vi "Log_heading-replay_v1.vi"() -> ()   [LabVIEW 2019]
panel:
  out "2D Picture 2":picture
  in  "file path":path
  out "Waveform Graph":dbl[](graph)
  out "array":dbl[](array[numeric])
  out "wgs84 graph":cluster{"X":dbl, "Y":dbl}[](graph)=[{"X"=4531061.36242506, "Y"=6178441.986275759}, {"X"=4531061.095248447, "Y"=6178442.06681065}, {"X"=4531060.929819513, "Y"=6178442.13471346}, {"X"=4531060.832518823, "Y"=6178442.197541265}, {"X"=4531060.770616335, "Y"=6178442.272890285}, {"X"=4531060.789204832, "Y"=6178442.28919004}, {"X"=4531060.772395123, "Y"=6178442.292968577}, {"X"=4531060.722855385, "Y"=6178442.314343328}, {"X"=4531060.606076811, "Y"=6178442.350832218}, {"X"=4531060.439758502, "Y"=6178442.40869586}, {"X"=4531060.290249909, "Y"=6178442.462780965}, {"X"=4531060.272550807, "Y"=6178442.456520356}, {"X"=4531060.239820785, "Y"=6178442.474116567}, {"X"=4531060.192059842, "Y"=6178442.5155695975}, {"X"=4531059.864759631, "Y"=6178442.691531702}, {"X"=4531059.779821708, "Y"=6178442.700385227}, {"X"=4531059.660374976, "Y"=6178442.7067566775}, {"X"=4531059.540038856, "Y"=6178442.7030889895}, {"X"=4531059.436512438, "Y"=6178442.695642762}, {"X"=4531059.299366613, "Y"=6178442.695753609}, {"X"=4531059.242711737, "Y"=6178442.6368152285}, {"X"=4531059.155105636, "Y"=6178442.615551336}, {"X"=4531059.104676525, "Y"=6178442.626886936}, {"X"=4531059.137406536, "Y"=6178442.609290733}, {"X"=4531059.171025946, "Y"=6178442.601733663}, {"X"=4531059.187835644, "Y"=6178442.597955129}, {"X"=4531059.189614435, "Y"=6178442.618033409}, {"X"=4531059.194950805, "Y"=6178442.678268249}, {"X"=4531059.527676117, "Y"=6178442.757063225}, {"X"=4531059.803746564, "Y"=6178442.776919831}, {"X"=4531059.710892868, "Y"=6178442.889943297}, {"X"=4531059.54190642, "Y"=6178442.917689476}, {"X"=4531059.377366953, "Y"=6178442.995631349}, {"X"=4531059.319911462, "Y"=6178443.121176009}, {"X"=4531058.873164632, "Y"=6178443.303509431}, {"X"=4531058.264546617, "Y"=6178443.593902031}, {"X"=4531057.714273541, "Y"=6178443.768789094}, {"X"=4531056.857868471, "Y"=6178443.971533049}, {"X"=4531055.882016951, "Y"=6178444.180648344}, {"X"=4531054.316047871, "Y"=6178444.501933605}, {"X"=4531053.000445728, "Y"=6178444.746462661}, {"X"=4531051.687423223, "Y"=6178444.826587329}, {"X"=4531050.336334684, "Y"=6178444.864073566}, {"X"=4531049.315213942, "Y"=6178444.755715789}, {"X"=4531048.093266786, "Y"=6178444.702739513}, {"X"=4531047.005797124, "Y"=6178444.619535221}, {"X"=4531046.041331673, "Y"=6178444.570115978}, {"X"=4531045.022790559, "Y"=6178444.297354844}, {"X"=4531044.25817308, "Y"=6178443.987994255}, {"X"=4531042.963740925, "Y"=6178444.084419535}, {"X"=4531041.977219151, "Y"=6178444.173065893}, {"X"=4531040.82438002, "Y"=6178444.319575647}, {"X"=4531039.649394999, "Y"=6178444.409629484}, {"X"=4531038.509808348, "Y"=6178444.512204443}, {"X"=4531037.261359377, "Y"=6178444.547098991}, {"X"=4531036.311926155, "Y"=6178444.473824003}, {"X"=4531035.260745918, "Y"=6178444.41318121}, {"X"=4531033.905213919, "Y"=6178444.400473842}, {"X"=4531032.472749636, "Y"=6178444.486971602}, {"X"=4531031.387061386, "Y"=6178444.423847185}, {"X"=4531030.066928328, "Y"=6178444.42366126}, {"X"=4531029.049278559, "Y"=6178444.16094189}, {"X"=4531027.591021638, "Y"=6178443.95630831}, {"X"=4531026.079757724, "Y"=6178443.927413569}, {"X"=4531024.871066671, "Y"=6178443.830505573}, {"X"=4531023.563297236, "Y"=6178443.77634695}, {"X"=4531022.521812914, "Y"=6178443.631615039}, {"X"=4531021.367998429, "Y"=6178443.573567053}, {"X"=4531020.007132588, "Y"=6178443.500627522}, {"X"=4531018.452557386, "Y"=6178443.563381526}, {"X"=4531016.914792171, "Y"=6178443.622357118}, {"X"=4531015.791039957, "Y"=6178443.516596719}, {"X"=4531014.692901826, "Y"=6178443.312928568}, {"X"=4531013.452372559, "Y"=6178443.243657234}, {"X"=4531012.218959265, "Y"=6178443.2546979}, {"X"=4531010.736961054, "Y"=6178443.362572499}, {"X"=4531009.554067381, "Y"=6178443.556796684}, {"X"=4531008.330439165, "Y"=6178443.678266158}, {"X"=4531007.172270388, "Y"=6178443.764543629}, {"X"=4531006.182197059, "Y"=6178443.813035869}, {"X"=4531004.925749518, "Y"=6178443.757582804}, {"X"=4531003.509212434, "Y"=6178443.830265695}, {"X"=4531002.303193948, "Y"=6178443.763477351}, {"X"=4531001.0052135065, "Y"=6178443.819749711}, {"X"=4530999.847845012, "Y"=6178443.721548208}, {"X"=4530998.599222504, "Y"=6178443.367409869}, {"X"=4530997.372746514, "Y"=6178443.069726953}, {"X"=4530996.291420466, "Y"=6178442.862283204}, {"X"=4530995.270216481, "Y"=6178442.559414194}, {"X"=4530994.338396943, "Y"=6178442.297886271}, {"X"=4530993.687891098, "Y"=6178441.921928868}, {"X"=4530993.020575724, "Y"=6178441.549750173}, {"X"=4530992.446202746, "Y"=6178441.259068059}, {"X"=4530991.660331448, "Y"=6178440.903300595}, {"X"=4530990.862987714, "Y"=6178440.61154533}, {"X"=4530989.863930333, "Y"=6178440.365132826}, {"X"=4530988.785181954, "Y"=6178439.993290142}, {"X"=4530987.896674796, "Y"=6178439.640117105}, {"X"=4530987.016081899, "Y"=6178439.182776809}, {"X"=4530986.158525055, "Y"=6178438.791930499}, {"X"=4530985.322133756, "Y"=6178438.252982851}, {"X"=4530984.685768332, "Y"=6178437.843132436}, {"X"=4530984.103297727, "Y"=6178437.267584608}, {"X"=4530983.746466159, "Y"=6178436.723226662}, {"X"=4530983.743430932, "Y"=6178435.915040186}, {"X"=4530983.693525295, "Y"=6178435.158344908}, {"X"=4530983.556014049, "Y"=6178434.380386928}, {"X"=4530983.381325537, "Y"=6178433.569830535}, {"X"=4530983.004923267, "Y"=6178432.804617277}, {"X"=4530982.739960196, "Y"=6178431.942681698}, {"X"=4530982.790020886, "Y"=6178431.1532757515}, {"X"=4530982.649042446, "Y"=6178430.529679693}, {"X"=4530982.459322566, "Y"=6178429.742979693}, {"X"=4530982.320920433, "Y"=6178428.954982738}, {"X"=4530982.173622549, "Y"=6178428.0665968135}, {"X"=4530981.62823454, "Y"=6178427.329131322}, {"X"=4530981.438513815, "Y"=6178426.54243141}, {"X"=4530981.246124193, "Y"=6178425.725614818}, {"X"=4530981.223608197, "Y"=6178424.89108958}, {"X"=4530981.094100545, "Y"=6178424.203481528}, {"X"=4530980.915053897, "Y"=6178423.537248316}, {"X"=4530981.074865304, "Y"=6178422.825558664}, {"X"=4530981.669943885, "Y"=6178421.995545852}, {"X"=4530981.934170355, "Y"=6178421.301339371}, {"X"=4530982.416030478, "Y"=6178420.547971078}, {"X"=4530982.20603299, "Y"=6178419.919411453}, {"X"=4530982.59761853, "Y"=6178419.114663753}, {"X"=4530982.943223482, "Y"=6178418.371446361}, {"X"=4530983.023434869, "Y"=6178417.7288433835}, {"X"=4530983.0691375965, "Y"=6178417.083758783}, {"X"=4530983.532501486, "Y"=6178416.508607976}, {"X"=4530984.062121182, "Y"=6178415.71378513}, {"X"=4530984.575728308, "Y"=6178414.738261373}, {"X"=4530985.043354852, "Y"=6178413.824267901}, {"X"=4530985.719812219, "Y"=6178412.945240799}, {"X"=4530986.349399512, "Y"=6178412.117705096}, {"X"=4530986.909969615, "Y"=6178411.285206017}, {"X"=4530987.637838169, "Y"=6178410.5993987685}, {"X"=4530988.845269547, "Y"=6178409.908175884}, {"X"=4530990.169478464, "Y"=6178409.180462327}, {"X"=4530991.561908379, "Y"=6178408.642190958}, {"X"=4530992.899369467, "Y"=6178407.87054172}, {"X"=4530993.945731143, "Y"=6178407.102896896}, {"X"=4530995.245126048, "Y"=6178406.288609087}, {"X"=4530996.648047593, "Y"=6178405.481764915}, {"X"=4530997.913824367, "Y"=6178404.675033256}, {"X"=4530998.862888482, "Y"=6178403.970214601}, {"X"=4530999.767658552, "Y"=6178403.15248521}, {"X"=4531000.828163074, "Y"=6178402.350941164}, {"X"=4531001.817871174, "Y"=6178401.524355709}, {"X"=4531002.7430099705, "Y"=6178400.743001848}, {"X"=4531003.608027404, "Y"=6178400.057074705}, {"X"=4531004.825157088, "Y"=6178399.281753247}, {"X"=4531005.845816726, "Y"=6178398.41749089}, {"X"=4531006.73022056, "Y"=6178397.563380394}, {"X"=4531007.61640379, "Y"=6178396.729347373}, {"X"=4531008.417742332, "Y"=6178396.098689213}, {"X"=4531009.312821996, "Y"=6178395.365045503}, {"X"=4531010.308759668, "Y"=6178394.608728314}, {"X"=4531010.841941455, "Y"=6178393.854048861}, {"X"=4531011.543219663, "Y"=6178393.061580644}, {"X"=4531012.576335659, "Y"=6178392.337860493}, {"X"=4531013.4466002695, "Y"=6178391.517641876}, {"X"=4531014.00895371, "Y"=6178390.705207859}, {"X"=4531014.772226336, "Y"=6178390.031908954}, {"X"=4531015.669976403, "Y"=6178389.328378749}, {"X"=4531016.655240558, "Y"=6178388.451588911}, {"X"=4531017.595413627, "Y"=6178387.646369493}, {"X"=4531018.445404212, "Y"=6178386.9842916755}, {"X"=4531018.971563079, "Y"=6178386.343816914}, {"X"=4531019.59324242, "Y"=6178385.6204340765}, {"X"=4531020.280474299, "Y"=6178385.056378583}, {"X"=4531021.072029946, "Y"=6178384.315284261}, {"X"=4531021.529967807, "Y"=6178383.485363264}, {"X"=4531022.314406787, "Y"=6178382.663955374}, {"X"=4531023.2032625815, "Y"=6178381.860029902}, {"X"=4531024.23727163, "Y"=6178381.1463417495}, {"X"=4531024.742173449, "Y"=6178380.459447751}, {"X"=4531025.615999362, "Y"=6178379.679377978}, {"X"=4531026.621634371, "Y"=6178378.838958925}, {"X"=4531027.767974779, "Y"=6178378.038581567}, {"X"=4531028.709929959, "Y"=6178377.2534335395}, {"X"=4531029.719124331, "Y"=6178376.453169198}, {"X"=4531030.5036580935, "Y"=6178375.826279149}, {"X"=4531031.516411452, "Y"=6178375.066170328}, {"X"=4531032.342478642, "Y"=6178374.327551261}, {"X"=4531033.658790734, "Y"=6178373.7039818335}, {"X"=4531035.2352562575, "Y"=6178373.114079729}, {"X"=4531036.86571019, "Y"=6178372.552996834}, {"X"=4531038.35555227, "Y"=6178372.146394164}, {"X"=4531039.811775328, "Y"=6178371.747349183}, {"X"=4531041.074288043, "Y"=6178371.484004215}, {"X"=4531042.657966306, "Y"=6178371.168936872}, {"X"=4531043.966553982, "Y"=6178371.038582218}, {"X"=4531045.505234291, "Y"=6178370.989610227}, {"X"=4531046.940387374, "Y"=6178370.933194681}, {"X"=4531048.287043757, "Y"=6178370.845478166}, {"X"=4531049.462136587, "Y"=6178370.949918508}, {"X"=4531050.707137665, "Y"=6178371.069360725}, {"X"=4531051.925636092, "Y"=6178371.276674773}, {"X"=4531053.001649715, "Y"=6178371.423868022}, {"X"=4531054.063522423, "Y"=6178371.604958085}, {"X"=4531055.343923036, "Y"=6178371.73692166}, {"X"=4531056.731409991, "Y"=6178371.916486175}, {"X"=4531057.948130019, "Y"=6178372.103723062}, {"X"=4531059.2674884265, "Y"=6178372.288364829}, {"X"=4531060.41163191, "Y"=6178372.4304827275}, {"X"=4531061.5637817625, "Y"=6178372.662953975}, {"X"=4531062.82390746, "Y"=6178372.95306562}, {"X"=4531064.037069952, "Y"=6178373.100146859}, {"X"=4531065.249343056, "Y"=6178373.237189062}, {"X"=4531066.432444453, "Y"=6178373.4319857}, {"X"=4531067.647386592, "Y"=6178373.599146142}, {"X"=4531068.807543307, "Y"=6178373.921972353}, {"X"=4531069.985399526, "Y"=6178374.251059206}, {"X"=4531071.112826171, "Y"=6178374.591483286}, {"X"=4531072.362278149, "Y"=6178374.761126214}, {"X"=4531073.548938524, "Y"=6178374.996081617}, {"X"=4531074.734709472, "Y"=6178375.220998018}, {"X"=4531075.988518144, "Y"=6178375.2463128045}, {"X"=4531077.323799403, "Y"=6178375.417140541}, {"X"=4531078.632577418, "Y"=6178375.675840814}, {"X"=4531079.936018335, "Y"=6178375.874305648}, {"X"=4531081.3721596515, "Y"=6178376.0224605715}, {"X"=4531082.628729365, "Y"=6178376.27242007}, {"X"=4531083.877384625, "Y"=6178376.626551941}, {"X"=4531085.0180641785, "Y"=6178376.923043358}, {"X"=4531086.153406647, "Y"=6178377.159299181}, {"X"=4531086.974697717, "Y"=6178377.527591075}, {"X"=4531087.4545440385, "Y"=6178378.105752066}, {"X"=4531088.40141923, "Y"=6178378.343419691}, {"X"=4531089.834003558, "Y"=6178378.451419775}, {"X"=4531091.277262362, "Y"=6178378.67989211}, {"X"=4531092.574568948, "Y"=6178379.0026112255}, {"X"=4531093.840833539, "Y"=6178379.168480203}, {"X"=4531095.048662892, "Y"=6178379.25533212}, {"X"=4531095.938083443, "Y"=6178379.618549757}, {"X"=4531096.926584712, "Y"=6178379.939015398}, {"X"=4531098.373402462, "Y"=6178380.207647139}, {"X"=4531099.6042688675, "Y"=6178380.360996598}, {"X"=4531100.833356456, "Y"=6178380.494267572}, {"X"=4531102.114653141, "Y"=6178380.63628074}, {"X"=4531103.531319355, "Y"=6178380.758102154}, {"X"=4531104.69939403, "Y"=6178380.97676513}, {"X"=4531105.671885175, "Y"=6178381.116523916}, {"X"=4531106.82137114, "Y"=6178381.318887517}, {"X"=4531108.565433378, "Y"=6178381.45926503}, {"X"=4531110.451801206, "Y"=6178381.270711307}, {"X"=4531112.307218145, "Y"=6178381.119833651}, {"X"=4531114.310367992, "Y"=6178380.8947881535}, {"X"=4531116.179927931, "Y"=6178380.710013429}, {"X"=4531117.915008334, "Y"=6178380.555470101}, {"X"=4531119.4837679025, "Y"=6178380.458794905}, {"X"=4531121.222407262, "Y"=6178380.344409419}, {"X"=4531123.170683199, "Y"=6178380.080503614}, {"X"=4531124.669535756, "Y"=6178379.968825969}, {"X"=4531126.092343553, "Y"=6178379.966398067}, {"X"=4531127.391255065, "Y"=6178379.92014661}, {"X"=4531128.363659995, "Y"=6178379.865379146}, {"X"=4531129.900581387, "Y"=6178379.7963412525}, {"X"=4531131.0968544325, "Y"=6178379.752684653}, {"X"=4531132.079133352, "Y"=6178380.002880428}, {"X"=4531133.501053443, "Y"=6178379.990413857}, {"X"=4531134.7982770335, "Y"=6178380.118613123}, {"X"=4531135.797366396, "Y"=6178380.365030662}, {"X"=4531137.091032587, "Y"=6178380.453072453}, {"X"=4531138.366999476, "Y"=6178380.534853874}, {"X"=4531139.581952214, "Y"=6178380.702027647}, {"X"=4531140.701291988, "Y"=6178380.757582756}, {"X"=4531141.9710335145, "Y"=6178380.769088216}, {"X"=4531143.468201078, "Y"=6178380.831862938}, {"X"=4531145.047640736, "Y"=6178380.85566426}, {"X"=4531146.485484407, "Y"=6178380.829380992}, {"X"=4531148.187932283, "Y"=6178380.886967416}, {"X"=4531149.763815479, "Y"=6178380.870611242}, {"X"=4531150.981349615, "Y"=6178380.873375337}, {"X"=4531152.508581932, "Y"=6178380.888435311}, {"X"=4531154.135697515, "Y"=6178380.676252104}, {"X"=4531155.785938228, "Y"=6178380.725097228}, {"X"=4531158.006835585, "Y"=6178380.635419734}, {"X"=4531159.500449378, "Y"=6178380.658038273}, {"X"=4531160.778287833, "Y"=6178380.954432427}, {"X"=4531162.149872312, "Y"=6178381.147836851}, {"X"=4531163.841739914, "Y"=6178381.27948173}, {"X"=4531165.326637487, "Y"=6178381.59076749}, {"X"=4531166.717701023, "Y"=6178381.8105128035}, {"X"=4531168.529821052, "Y"=6178381.751294012}, {"X"=4531169.835055363, "Y"=6178381.969855328}, {"X"=4531170.320948598, "Y"=6178382.229250287}, {"X"=4531171.080252015, "Y"=6178382.478380797}, {"X"=4531171.576016277, "Y"=6178383.042742996}, {"X"=4531172.72035149, "Y"=6178383.573942711}, {"X"=4531174.0849103825, "Y"=6178383.88156489}, {"X"=4531175.150355192, "Y"=6178384.102834543}, {"X"=4531175.369952878, "Y"=6178384.452811636}, {"X"=4531175.2817180995, "Y"=6178385.005102757}, {"X"=4531174.792706191, "Y"=6178385.678205996}, {"X"=4531174.569187919, "Y"=6178386.445219818}, {"X"=4531173.566174453, "Y"=6178387.315784675}, {"X"=4531173.004585712, "Y"=6178387.943764852}, {"X"=4531172.677538117, "Y"=6178388.703332222}, {"X"=4531172.19386255, "Y"=6178389.436671552}, {"X"=4531171.71018701, "Y"=6178390.170010573}, {"X"=4531171.741401999, "Y"=6178390.715927548}, {"X"=4531171.907987807, "Y"=6178391.2416532375}, {"X"=4531171.572046452, "Y"=6178391.90082367}, {"X"=4531171.167085634, "Y"=6178392.555030101}, {"X"=4531171.157652611, "Y"=6178393.222718802}, {"X"=4531170.708486615, "Y"=6178393.958538462}, {"X"=4531169.790414286, "Y"=6178394.820244326}, {"X"=4531169.3456951305, "Y"=6178395.606261164}, {"X"=4531168.858462186, "Y"=6178396.299439562}, {"X"=4531168.570283294, "Y"=6178396.917153108}, {"X"=4531168.074244299, "Y"=6178397.70446596}, {"X"=4531167.710907955, "Y"=6178398.441468852}, {"X"=4531167.532396106, "Y"=6178398.942374006}, {"X"=4531167.076115536, "Y"=6178399.597874829}, {"X"=4531166.6110288715, "Y"=6178400.347510266}, {"X"=4531166.296344272, "Y"=6178401.053096698}, {"X"=4531165.944482004, "Y"=6178401.726082247}, {"X"=4531165.362526449, "Y"=6178402.317677534}, {"X"=4531164.53900361, "Y"=6178402.891898637}, {"X"=4531163.9013690315, "Y"=6178403.629122646}, {"X"=4531163.401685826, "Y"=6178404.181744099}, {"X"=4531163.1179536, "Y"=6178404.849652828}, {"X"=4531162.782901618, "Y"=6178405.518858123}, {"X"=4531162.6849701125, "Y"=6178406.155239621}, {"X"=4531162.467588969, "Y"=6178406.7979932325}, {"X"=4531161.8820765605, "Y"=6178407.349428364}, {"X"=4531161.4178794585, "Y"=6178408.109100074}, {"X"=4531161.144818966, "Y"=6178408.897482027}, {"X"=4531160.637306067, "Y"=6178409.748805623}, {"X"=4531159.989976334, "Y"=6178410.570121538}, {"X"=4531159.336421459, "Y"=6178411.321160347}, {"X"=4531158.668724526, "Y"=6178412.10609606}, {"X"=4531158.485939669, "Y"=6178412.9458595095}, {"X"=4531157.989901085, "Y"=6178413.733165388}, {"X"=4531157.419594476, "Y"=6178414.6497991355}, {"X"=4531157.043894533, "Y"=6178415.440771885}, {"X"=4531156.463892334, "Y"=6178416.441499566}, {"X"=4531155.611371523, "Y"=6178417.462527762}, {"X"=4531155.200359533, "Y"=6178418.435506958}, {"X"=4531154.830884667, "Y"=6178419.296754719}, {"X"=4531154.30211532, "Y"=6178420.101654765}, {"X"=4531153.473432615, "Y"=6178421.004688968}, {"X"=4531152.974726329, "Y"=6178421.761872893}, {"X"=4531152.53801116, "Y"=6178422.638233842}, {"X"=4531152.18712486, "Y"=6178423.515780127}, {"X"=4531151.659244953, "Y"=6178424.330717752}, {"X"=4531150.965932405, "Y"=6178425.21355987}, {"X"=4531150.225746978, "Y"=6178426.1478953}, {"X"=4531149.141357127, "Y"=6178427.067447557}, {"X"=4531148.517953012, "Y"=6178427.965291934}, {"X"=4531147.82019449, "Y"=6178428.797934613}, {"X"=4531147.213600552, "Y"=6178429.691999431}, {"X"=4531146.807837723, "Y"=6178430.5306810085}, {"X"=4531146.549005081, "Y"=6178431.4796857955}, {"X"=4531146.207814394, "Y"=6178432.27313397}, {"X"=4531145.821442939, "Y"=6178432.943626221}, {"X"=4531145.026295356, "Y"=6178433.644567707}, {"X"=4531144.401112979, "Y"=6178434.522329833}, {"X"=4531143.8157756375, "Y"=6178435.462810415}, {"X"=4531142.856085532, "Y"=6178436.241694084}, {"X"=4531141.712202374, "Y"=6178436.683125389}, {"X"=4531140.460345346, "Y"=6178437.066912421}, {"X"=4531138.7855711365, "Y"=6178437.515045113}, {"X"=4531137.2540838905, "Y"=6178437.8388156835}, {"X"=4531135.901281937, "Y"=6178438.050746028}, {"X"=4531134.513081851, "Y"=6178438.250154628}, {"X"=4531133.302677512, "Y"=6178438.327683812}, {"X"=4531131.97727157, "Y"=6178438.461781153}, {"X"=4531130.434225819, "Y"=6178438.655039164}, {"X"=4531128.833636347, "Y"=6178438.779317742}, {"X"=4531127.188842603, "Y"=6178438.985207698}, {"X"=4531125.765159796, "Y"=6178438.977567875}, {"X"=4531124.333560398, "Y"=6178439.074100451}, {"X"=4531123.178034697, "Y"=6178439.19049111}, {"X"=4531121.688891792, "Y"=6178439.218044568}, {"X"=4531120.143983659, "Y"=6178439.196697701}, {"X"=4531118.777846783, "Y"=6178439.258037677}, {"X"=4531117.273760713, "Y"=6178439.503974881}, {"X"=4531115.719158377, "Y"=6178439.566721672}, {"X"=4531114.359247835, "Y"=6178439.698337167}, {"X"=4531112.978970496, "Y"=6178439.793573919}, {"X"=4531111.604831579, "Y"=6178439.764560291}, {"X"=4531110.167010706, "Y"=6178439.790818312}, {"X"=4531108.717716249, "Y"=6178439.881090899}, {"X"=4531107.251612302, "Y"=6178439.975142099}, {"X"=4531105.856218201, "Y"=6178439.899711062}, {"X"=4531104.335238762, "Y"=6178439.954901642}, {"X"=4531102.807232527, "Y"=6178440.124303117}, {"X"=4531101.328766988, "Y"=6178440.272329651}, {"X"=4531099.891838069, "Y"=6178440.308627729}, {"X"=4531098.531042268, "Y"=6178440.430204515}, {"X"=4531097.2551853685, "Y"=6178440.542927866}, {"X"=4531095.906753391, "Y"=6178440.610529815}, {"X"=4531094.453905393, "Y"=6178440.660646058}, {"X"=4531093.051487248, "Y"=6178440.699426771}, {"X"=4531091.507563893, "Y"=6178440.882646296}, {"X"=4531090.124624367, "Y"=6178440.947766378}, {"X"=4531088.636379567, "Y"=6178440.985361588}, {"X"=4531086.920802104, "Y"=6178441.166209676}, {"X"=4531085.168048208, "Y"=6178441.314457928}, {"X"=4531083.614256263, "Y"=6178441.1927222395}, {"X"=4531082.135708063, "Y"=6178441.1462256685}, {"X"=4531080.787191631, "Y"=6178441.019304884}, {"X"=4531079.550118306, "Y"=6178440.795660042}, {"X"=4531078.355558375, "Y"=6178440.664850496}, {"X"=4531077.03630355, "Y"=6178440.674700762}, {"X"=4531075.614411686, "Y"=6178440.68714403}, {"X"=4531074.112918239, "Y"=6178440.7686761385}, {"X"=4531072.594615453, "Y"=6178440.853986876}, {"X"=4531071.1807291135, "Y"=6178440.956783168}, {"X"=4531069.776626355, "Y"=6178441.170010469}, {"X"=4531068.367187707, "Y"=6178441.323002671}, {"X"=4531067.229284766, "Y"=6178441.251132974}, {"X"=4531066.229328779, "Y"=6178440.994669049}, {"X"=4531065.468266617, "Y"=6178440.725462372}, {"X"=4531065.011647067, "Y"=6178440.602842985}, {"X"=4531064.836523361, "Y"=6178440.754837769}, {"X"=4531064.734775603, "Y"=6178440.767469879}, {"X"=4531064.70204554, "Y"=6178440.7850661315}, {"X"=4531064.7259704, "Y"=6178440.861600875}, {"X"=4531064.616306829, "Y"=6178440.978403134}, {"X"=4531064.571213997, "Y"=6178441.049973729}, {"X"=4531064.4960592715, "Y"=6178441.16925804}, {"X"=4531064.430599156, "Y"=6178441.204450528}, {"X"=4531064.349218701, "Y"=6178441.253460727}, {"X"=4531064.235997578, "Y"=6178441.330106311}, {"X"=4531064.123665855, "Y"=6178441.41679105}, {"X"=4531064.026365073, "Y"=6178441.479618935}, {"X"=4531064.015781082, "Y"=6178441.553671578}, {"X"=4531064.05562626, "Y"=6178441.616388603}]
  in  "dt":u32=1
  out "utm graph":cluster{"X":dbl, "Y":dbl}[](graph)=[{"X"=4531061.36242506, "Y"=6178441.986275759}, {"X"=4531061.095248447, "Y"=6178442.06681065}, {"X"=4531060.929819513, "Y"=6178442.13471346}, {"X"=4531060.832518823, "Y"=6178442.197541265}, {"X"=4531060.770616335, "Y"=6178442.272890285}, {"X"=4531060.789204832, "Y"=6178442.28919004}, {"X"=4531060.772395123, "Y"=6178442.292968577}, {"X"=4531060.722855385, "Y"=6178442.314343328}, {"X"=4531060.606076811, "Y"=6178442.350832218}, {"X"=4531060.439758502, "Y"=6178442.40869586}, {"X"=4531060.290249909, "Y"=6178442.462780965}, {"X"=4531060.272550807, "Y"=6178442.456520356}, {"X"=4531060.239820785, "Y"=6178442.474116567}, {"X"=4531060.192059842, "Y"=6178442.5155695975}, {"X"=4531059.864759631, "Y"=6178442.691531702}, {"X"=4531059.779821708, "Y"=6178442.700385227}, {"X"=4531059.660374976, "Y"=6178442.7067566775}, {"X"=4531059.540038856, "Y"=6178442.7030889895}, {"X"=4531059.436512438, "Y"=6178442.695642762}, {"X"=4531059.299366613, "Y"=6178442.695753609}, {"X"=4531059.242711737, "Y"=6178442.6368152285}, {"X"=4531059.155105636, "Y"=6178442.615551336}, {"X"=4531059.104676525, "Y"=6178442.626886936}, {"X"=4531059.137406536, "Y"=6178442.609290733}, {"X"=4531059.171025946, "Y"=6178442.601733663}, {"X"=4531059.187835644, "Y"=6178442.597955129}, {"X"=4531059.189614435, "Y"=6178442.618033409}, {"X"=4531059.194950805, "Y"=6178442.678268249}, {"X"=4531059.527676117, "Y"=6178442.757063225}, {"X"=4531059.803746564, "Y"=6178442.776919831}, {"X"=4531059.710892868, "Y"=6178442.889943297}, {"X"=4531059.54190642, "Y"=6178442.917689476}, {"X"=4531059.377366953, "Y"=6178442.995631349}, {"X"=4531059.319911462, "Y"=6178443.121176009}, {"X"=4531058.873164632, "Y"=6178443.303509431}, {"X"=4531058.264546617, "Y"=6178443.593902031}, {"X"=4531057.714273541, "Y"=6178443.768789094}, {"X"=4531056.857868471, "Y"=6178443.971533049}, {"X"=4531055.882016951, "Y"=6178444.180648344}, {"X"=4531054.316047871, "Y"=6178444.501933605}, {"X"=4531053.000445728, "Y"=6178444.746462661}, {"X"=4531051.687423223, "Y"=6178444.826587329}, {"X"=4531050.336334684, "Y"=6178444.864073566}, {"X"=4531049.315213942, "Y"=6178444.755715789}, {"X"=4531048.093266786, "Y"=6178444.702739513}, {"X"=4531047.005797124, "Y"=6178444.619535221}, {"X"=4531046.041331673, "Y"=6178444.570115978}, {"X"=4531045.022790559, "Y"=6178444.297354844}, {"X"=4531044.25817308, "Y"=6178443.987994255}, {"X"=4531042.963740925, "Y"=6178444.084419535}, {"X"=4531041.977219151, "Y"=6178444.173065893}, {"X"=4531040.82438002, "Y"=6178444.319575647}, {"X"=4531039.649394999, "Y"=6178444.409629484}, {"X"=4531038.509808348, "Y"=6178444.512204443}, {"X"=4531037.261359377, "Y"=6178444.547098991}, {"X"=4531036.311926155, "Y"=6178444.473824003}, {"X"=4531035.260745918, "Y"=6178444.41318121}, {"X"=4531033.905213919, "Y"=6178444.400473842}, {"X"=4531032.472749636, "Y"=6178444.486971602}, {"X"=4531031.387061386, "Y"=6178444.423847185}, {"X"=4531030.066928328, "Y"=6178444.42366126}, {"X"=4531029.049278559, "Y"=6178444.16094189}, {"X"=4531027.591021638, "Y"=6178443.95630831}, {"X"=4531026.079757724, "Y"=6178443.927413569}, {"X"=4531024.871066671, "Y"=6178443.830505573}, {"X"=4531023.563297236, "Y"=6178443.77634695}, {"X"=4531022.521812914, "Y"=6178443.631615039}, {"X"=4531021.367998429, "Y"=6178443.573567053}, {"X"=4531020.007132588, "Y"=6178443.500627522}, {"X"=4531018.452557386, "Y"=6178443.563381526}, {"X"=4531016.914792171, "Y"=6178443.622357118}, {"X"=4531015.791039957, "Y"=6178443.516596719}, {"X"=4531014.692901826, "Y"=6178443.312928568}, {"X"=4531013.452372559, "Y"=6178443.243657234}, {"X"=4531012.218959265, "Y"=6178443.2546979}, {"X"=4531010.736961054, "Y"=6178443.362572499}, {"X"=4531009.554067381, "Y"=6178443.556796684}, {"X"=4531008.330439165, "Y"=6178443.678266158}, {"X"=4531007.172270388, "Y"=6178443.764543629}, {"X"=4531006.182197059, "Y"=6178443.813035869}, {"X"=4531004.925749518, "Y"=6178443.757582804}, {"X"=4531003.509212434, "Y"=6178443.830265695}, {"X"=4531002.303193948, "Y"=6178443.763477351}, {"X"=4531001.0052135065, "Y"=6178443.819749711}, {"X"=4530999.847845012, "Y"=6178443.721548208}, {"X"=4530998.599222504, "Y"=6178443.367409869}, {"X"=4530997.372746514, "Y"=6178443.069726953}, {"X"=4530996.291420466, "Y"=6178442.862283204}, {"X"=4530995.270216481, "Y"=6178442.559414194}, {"X"=4530994.338396943, "Y"=6178442.297886271}, {"X"=4530993.687891098, "Y"=6178441.921928868}, {"X"=4530993.020575724, "Y"=6178441.549750173}, {"X"=4530992.446202746, "Y"=6178441.259068059}, {"X"=4530991.660331448, "Y"=6178440.903300595}, {"X"=4530990.862987714, "Y"=6178440.61154533}, {"X"=4530989.863930333, "Y"=6178440.365132826}, {"X"=4530988.785181954, "Y"=6178439.993290142}, {"X"=4530987.896674796, "Y"=6178439.640117105}, {"X"=4530987.016081899, "Y"=6178439.182776809}, {"X"=4530986.158525055, "Y"=6178438.791930499}, {"X"=4530985.322133756, "Y"=6178438.252982851}, {"X"=4530984.685768332, "Y"=6178437.843132436}, {"X"=4530984.103297727, "Y"=6178437.267584608}, {"X"=4530983.746466159, "Y"=6178436.723226662}, {"X"=4530983.743430932, "Y"=6178435.915040186}, {"X"=4530983.693525295, "Y"=6178435.158344908}, {"X"=4530983.556014049, "Y"=6178434.380386928}, {"X"=4530983.381325537, "Y"=6178433.569830535}, {"X"=4530983.004923267, "Y"=6178432.804617277}, {"X"=4530982.739960196, "Y"=6178431.942681698}, {"X"=4530982.790020886, "Y"=6178431.1532757515}, {"X"=4530982.649042446, "Y"=6178430.529679693}, {"X"=4530982.459322566, "Y"=6178429.742979693}, {"X"=4530982.320920433, "Y"=6178428.954982738}, {"X"=4530982.173622549, "Y"=6178428.0665968135}, {"X"=4530981.62823454, "Y"=6178427.329131322}, {"X"=4530981.438513815, "Y"=6178426.54243141}, {"X"=4530981.246124193, "Y"=6178425.725614818}, {"X"=4530981.223608197, "Y"=6178424.89108958}, {"X"=4530981.094100545, "Y"=6178424.203481528}, {"X"=4530980.915053897, "Y"=6178423.537248316}, {"X"=4530981.074865304, "Y"=6178422.825558664}, {"X"=4530981.669943885, "Y"=6178421.995545852}, {"X"=4530981.934170355, "Y"=6178421.301339371}, {"X"=4530982.416030478, "Y"=6178420.547971078}, {"X"=4530982.20603299, "Y"=6178419.919411453}, {"X"=4530982.59761853, "Y"=6178419.114663753}, {"X"=4530982.943223482, "Y"=6178418.371446361}, {"X"=4530983.023434869, "Y"=6178417.7288433835}, {"X"=4530983.0691375965, "Y"=6178417.083758783}, {"X"=4530983.532501486, "Y"=6178416.508607976}, {"X"=4530984.062121182, "Y"=6178415.71378513}, {"X"=4530984.575728308, "Y"=6178414.738261373}, {"X"=4530985.043354852, "Y"=6178413.824267901}, {"X"=4530985.719812219, "Y"=6178412.945240799}, {"X"=4530986.349399512, "Y"=6178412.117705096}, {"X"=4530986.909969615, "Y"=6178411.285206017}, {"X"=4530987.637838169, "Y"=6178410.5993987685}, {"X"=4530988.845269547, "Y"=6178409.908175884}, {"X"=4530990.169478464, "Y"=6178409.180462327}, {"X"=4530991.561908379, "Y"=6178408.642190958}, {"X"=4530992.899369467, "Y"=6178407.87054172}, {"X"=4530993.945731143, "Y"=6178407.102896896}, {"X"=4530995.245126048, "Y"=6178406.288609087}, {"X"=4530996.648047593, "Y"=6178405.481764915}, {"X"=4530997.913824367, "Y"=6178404.675033256}, {"X"=4530998.862888482, "Y"=6178403.970214601}, {"X"=4530999.767658552, "Y"=6178403.15248521}, {"X"=4531000.828163074, "Y"=6178402.350941164}, {"X"=4531001.817871174, "Y"=6178401.524355709}, {"X"=4531002.7430099705, "Y"=6178400.743001848}, {"X"=4531003.608027404, "Y"=6178400.057074705}, {"X"=4531004.825157088, "Y"=6178399.281753247}, {"X"=4531005.845816726, "Y"=6178398.41749089}, {"X"=4531006.73022056, "Y"=6178397.563380394}, {"X"=4531007.61640379, "Y"=6178396.729347373}, {"X"=4531008.417742332, "Y"=6178396.098689213}, {"X"=4531009.312821996, "Y"=6178395.365045503}, {"X"=4531010.308759668, "Y"=6178394.608728314}, {"X"=4531010.841941455, "Y"=6178393.854048861}, {"X"=4531011.543219663, "Y"=6178393.061580644}, {"X"=4531012.576335659, "Y"=6178392.337860493}, {"X"=4531013.4466002695, "Y"=6178391.517641876}, {"X"=4531014.00895371, "Y"=6178390.705207859}, {"X"=4531014.772226336, "Y"=6178390.031908954}, {"X"=4531015.669976403, "Y"=6178389.328378749}, {"X"=4531016.655240558, "Y"=6178388.451588911}, {"X"=4531017.595413627, "Y"=6178387.646369493}, {"X"=4531018.445404212, "Y"=6178386.9842916755}, {"X"=4531018.971563079, "Y"=6178386.343816914}, {"X"=4531019.59324242, "Y"=6178385.6204340765}, {"X"=4531020.280474299, "Y"=6178385.056378583}, {"X"=4531021.072029946, "Y"=6178384.315284261}, {"X"=4531021.529967807, "Y"=6178383.485363264}, {"X"=4531022.314406787, "Y"=6178382.663955374}, {"X"=4531023.2032625815, "Y"=6178381.860029902}, {"X"=4531024.23727163, "Y"=6178381.1463417495}, {"X"=4531024.742173449, "Y"=6178380.459447751}, {"X"=4531025.615999362, "Y"=6178379.679377978}, {"X"=4531026.621634371, "Y"=6178378.838958925}, {"X"=4531027.767974779, "Y"=6178378.038581567}, {"X"=4531028.709929959, "Y"=6178377.2534335395}, {"X"=4531029.719124331, "Y"=6178376.453169198}, {"X"=4531030.5036580935, "Y"=6178375.826279149}, {"X"=4531031.516411452, "Y"=6178375.066170328}, {"X"=4531032.342478642, "Y"=6178374.327551261}, {"X"=4531033.658790734, "Y"=6178373.7039818335}, {"X"=4531035.2352562575, "Y"=6178373.114079729}, {"X"=4531036.86571019, "Y"=6178372.552996834}, {"X"=4531038.35555227, "Y"=6178372.146394164}, {"X"=4531039.811775328, "Y"=6178371.747349183}, {"X"=4531041.074288043, "Y"=6178371.484004215}, {"X"=4531042.657966306, "Y"=6178371.168936872}, {"X"=4531043.966553982, "Y"=6178371.038582218}, {"X"=4531045.505234291, "Y"=6178370.989610227}, {"X"=4531046.940387374, "Y"=6178370.933194681}, {"X"=4531048.287043757, "Y"=6178370.845478166}, {"X"=4531049.462136587, "Y"=6178370.949918508}, {"X"=4531050.707137665, "Y"=6178371.069360725}, {"X"=4531051.925636092, "Y"=6178371.276674773}, {"X"=4531053.001649715, "Y"=6178371.423868022}, {"X"=4531054.063522423, "Y"=6178371.604958085}, {"X"=4531055.343923036, "Y"=6178371.73692166}, {"X"=4531056.731409991, "Y"=6178371.916486175}, {"X"=4531057.948130019, "Y"=6178372.103723062}, {"X"=4531059.2674884265, "Y"=6178372.288364829}, {"X"=4531060.41163191, "Y"=6178372.4304827275}, {"X"=4531061.5637817625, "Y"=6178372.662953975}, {"X"=4531062.82390746, "Y"=6178372.95306562}, {"X"=4531064.037069952, "Y"=6178373.100146859}, {"X"=4531065.249343056, "Y"=6178373.237189062}, {"X"=4531066.432444453, "Y"=6178373.4319857}, {"X"=4531067.647386592, "Y"=6178373.599146142}, {"X"=4531068.807543307, "Y"=6178373.921972353}, {"X"=4531069.985399526, "Y"=6178374.251059206}, {"X"=4531071.112826171, "Y"=6178374.591483286}, {"X"=4531072.362278149, "Y"=6178374.761126214}, {"X"=4531073.548938524, "Y"=6178374.996081617}, {"X"=4531074.734709472, "Y"=6178375.220998018}, {"X"=4531075.988518144, "Y"=6178375.2463128045}, {"X"=4531077.323799403, "Y"=6178375.417140541}, {"X"=4531078.632577418, "Y"=6178375.675840814}, {"X"=4531079.936018335, "Y"=6178375.874305648}, {"X"=4531081.3721596515, "Y"=6178376.0224605715}, {"X"=4531082.628729365, "Y"=6178376.27242007}, {"X"=4531083.877384625, "Y"=6178376.626551941}, {"X"=4531085.0180641785, "Y"=6178376.923043358}, {"X"=4531086.153406647, "Y"=6178377.159299181}, {"X"=4531086.974697717, "Y"=6178377.527591075}, {"X"=4531087.4545440385, "Y"=6178378.105752066}, {"X"=4531088.40141923, "Y"=6178378.343419691}, {"X"=4531089.834003558, "Y"=6178378.451419775}, {"X"=4531091.277262362, "Y"=6178378.67989211}, {"X"=4531092.574568948, "Y"=6178379.0026112255}, {"X"=4531093.840833539, "Y"=6178379.168480203}, {"X"=4531095.048662892, "Y"=6178379.25533212}, {"X"=4531095.938083443, "Y"=6178379.618549757}, {"X"=4531096.926584712, "Y"=6178379.939015398}, {"X"=4531098.373402462, "Y"=6178380.207647139}, {"X"=4531099.6042688675, "Y"=6178380.360996598}, {"X"=4531100.833356456, "Y"=6178380.494267572}, {"X"=4531102.114653141, "Y"=6178380.63628074}, {"X"=4531103.531319355, "Y"=6178380.758102154}, {"X"=4531104.69939403, "Y"=6178380.97676513}, {"X"=4531105.671885175, "Y"=6178381.116523916}, {"X"=4531106.82137114, "Y"=6178381.318887517}, {"X"=4531108.565433378, "Y"=6178381.45926503}, {"X"=4531110.451801206, "Y"=6178381.270711307}, {"X"=4531112.307218145, "Y"=6178381.119833651}, {"X"=4531114.310367992, "Y"=6178380.8947881535}, {"X"=4531116.179927931, "Y"=6178380.710013429}, {"X"=4531117.915008334, "Y"=6178380.555470101}, {"X"=4531119.4837679025, "Y"=6178380.458794905}, {"X"=4531121.222407262, "Y"=6178380.344409419}, {"X"=4531123.170683199, "Y"=6178380.080503614}, {"X"=4531124.669535756, "Y"=6178379.968825969}, {"X"=4531126.092343553, "Y"=6178379.966398067}, {"X"=4531127.391255065, "Y"=6178379.92014661}, {"X"=4531128.363659995, "Y"=6178379.865379146}, {"X"=4531129.900581387, "Y"=6178379.7963412525}, {"X"=4531131.0968544325, "Y"=6178379.752684653}, {"X"=4531132.079133352, "Y"=6178380.002880428}, {"X"=4531133.501053443, "Y"=6178379.990413857}, {"X"=4531134.7982770335, "Y"=6178380.118613123}, {"X"=4531135.797366396, "Y"=6178380.365030662}, {"X"=4531137.091032587, "Y"=6178380.453072453}, {"X"=4531138.366999476, "Y"=6178380.534853874}, {"X"=4531139.581952214, "Y"=6178380.702027647}, {"X"=4531140.701291988, "Y"=6178380.757582756}, {"X"=4531141.9710335145, "Y"=6178380.769088216}, {"X"=4531143.468201078, "Y"=6178380.831862938}, {"X"=4531145.047640736, "Y"=6178380.85566426}, {"X"=4531146.485484407, "Y"=6178380.829380992}, {"X"=4531148.187932283, "Y"=6178380.886967416}, {"X"=4531149.763815479, "Y"=6178380.870611242}, {"X"=4531150.981349615, "Y"=6178380.873375337}, {"X"=4531152.508581932, "Y"=6178380.888435311}, {"X"=4531154.135697515, "Y"=6178380.676252104}, {"X"=4531155.785938228, "Y"=6178380.725097228}, {"X"=4531158.006835585, "Y"=6178380.635419734}, {"X"=4531159.500449378, "Y"=6178380.658038273}, {"X"=4531160.778287833, "Y"=6178380.954432427}, {"X"=4531162.149872312, "Y"=6178381.147836851}, {"X"=4531163.841739914, "Y"=6178381.27948173}, {"X"=4531165.326637487, "Y"=6178381.59076749}, {"X"=4531166.717701023, "Y"=6178381.8105128035}, {"X"=4531168.529821052, "Y"=6178381.751294012}, {"X"=4531169.835055363, "Y"=6178381.969855328}, {"X"=4531170.320948598, "Y"=6178382.229250287}, {"X"=4531171.080252015, "Y"=6178382.478380797}, {"X"=4531171.576016277, "Y"=6178383.042742996}, {"X"=4531172.72035149, "Y"=6178383.573942711}, {"X"=4531174.0849103825, "Y"=6178383.88156489}, {"X"=4531175.150355192, "Y"=6178384.102834543}, {"X"=4531175.369952878, "Y"=6178384.452811636}, {"X"=4531175.2817180995, "Y"=6178385.005102757}, {"X"=4531174.792706191, "Y"=6178385.678205996}, {"X"=4531174.569187919, "Y"=6178386.445219818}, {"X"=4531173.566174453, "Y"=6178387.315784675}, {"X"=4531173.004585712, "Y"=6178387.943764852}, {"X"=4531172.677538117, "Y"=6178388.703332222}, {"X"=4531172.19386255, "Y"=6178389.436671552}, {"X"=4531171.71018701, "Y"=6178390.170010573}, {"X"=4531171.741401999, "Y"=6178390.715927548}, {"X"=4531171.907987807, "Y"=6178391.2416532375}, {"X"=4531171.572046452, "Y"=6178391.90082367}, {"X"=4531171.167085634, "Y"=6178392.555030101}, {"X"=4531171.157652611, "Y"=6178393.222718802}, {"X"=4531170.708486615, "Y"=6178393.958538462}, {"X"=4531169.790414286, "Y"=6178394.820244326}, {"X"=4531169.3456951305, "Y"=6178395.606261164}, {"X"=4531168.858462186, "Y"=6178396.299439562}, {"X"=4531168.570283294, "Y"=6178396.917153108}, {"X"=4531168.074244299, "Y"=6178397.70446596}, {"X"=4531167.710907955, "Y"=6178398.441468852}, {"X"=4531167.532396106, "Y"=6178398.942374006}, {"X"=4531167.076115536, "Y"=6178399.597874829}, {"X"=4531166.6110288715, "Y"=6178400.347510266}, {"X"=4531166.296344272, "Y"=6178401.053096698}, {"X"=4531165.944482004, "Y"=6178401.726082247}, {"X"=4531165.362526449, "Y"=6178402.317677534}, {"X"=4531164.53900361, "Y"=6178402.891898637}, {"X"=4531163.9013690315, "Y"=6178403.629122646}, {"X"=4531163.401685826, "Y"=6178404.181744099}, {"X"=4531163.1179536, "Y"=6178404.849652828}, {"X"=4531162.782901618, "Y"=6178405.518858123}, {"X"=4531162.6849701125, "Y"=6178406.155239621}, {"X"=4531162.467588969, "Y"=6178406.7979932325}, {"X"=4531161.8820765605, "Y"=6178407.349428364}, {"X"=4531161.4178794585, "Y"=6178408.109100074}, {"X"=4531161.144818966, "Y"=6178408.897482027}, {"X"=4531160.637306067, "Y"=6178409.748805623}, {"X"=4531159.989976334, "Y"=6178410.570121538}, {"X"=4531159.336421459, "Y"=6178411.321160347}, {"X"=4531158.668724526, "Y"=6178412.10609606}, {"X"=4531158.485939669, "Y"=6178412.9458595095}, {"X"=4531157.989901085, "Y"=6178413.733165388}, {"X"=4531157.419594476, "Y"=6178414.6497991355}, {"X"=4531157.043894533, "Y"=6178415.440771885}, {"X"=4531156.463892334, "Y"=6178416.441499566}, {"X"=4531155.611371523, "Y"=6178417.462527762}, {"X"=4531155.200359533, "Y"=6178418.435506958}, {"X"=4531154.830884667, "Y"=6178419.296754719}, {"X"=4531154.30211532, "Y"=6178420.101654765}, {"X"=4531153.473432615, "Y"=6178421.004688968}, {"X"=4531152.974726329, "Y"=6178421.761872893}, {"X"=4531152.53801116, "Y"=6178422.638233842}, {"X"=4531152.18712486, "Y"=6178423.515780127}, {"X"=4531151.659244953, "Y"=6178424.330717752}, {"X"=4531150.965932405, "Y"=6178425.21355987}, {"X"=4531150.225746978, "Y"=6178426.1478953}, {"X"=4531149.141357127, "Y"=6178427.067447557}, {"X"=4531148.517953012, "Y"=6178427.965291934}, {"X"=4531147.82019449, "Y"=6178428.797934613}, {"X"=4531147.213600552, "Y"=6178429.691999431}, {"X"=4531146.807837723, "Y"=6178430.5306810085}, {"X"=4531146.549005081, "Y"=6178431.4796857955}, {"X"=4531146.207814394, "Y"=6178432.27313397}, {"X"=4531145.821442939, "Y"=6178432.943626221}, {"X"=4531145.026295356, "Y"=6178433.644567707}, {"X"=4531144.401112979, "Y"=6178434.522329833}, {"X"=4531143.8157756375, "Y"=6178435.462810415}, {"X"=4531142.856085532, "Y"=6178436.241694084}, {"X"=4531141.712202374, "Y"=6178436.683125389}, {"X"=4531140.460345346, "Y"=6178437.066912421}, {"X"=4531138.7855711365, "Y"=6178437.515045113}, {"X"=4531137.2540838905, "Y"=6178437.8388156835}, {"X"=4531135.901281937, "Y"=6178438.050746028}, {"X"=4531134.513081851, "Y"=6178438.250154628}, {"X"=4531133.302677512, "Y"=6178438.327683812}, {"X"=4531131.97727157, "Y"=6178438.461781153}, {"X"=4531130.434225819, "Y"=6178438.655039164}, {"X"=4531128.833636347, "Y"=6178438.779317742}, {"X"=4531127.188842603, "Y"=6178438.985207698}, {"X"=4531125.765159796, "Y"=6178438.977567875}, {"X"=4531124.333560398, "Y"=6178439.074100451}, {"X"=4531123.178034697, "Y"=6178439.19049111}, {"X"=4531121.688891792, "Y"=6178439.218044568}, {"X"=4531120.143983659, "Y"=6178439.196697701}, {"X"=4531118.777846783, "Y"=6178439.258037677}, {"X"=4531117.273760713, "Y"=6178439.503974881}, {"X"=4531115.719158377, "Y"=6178439.566721672}, {"X"=4531114.359247835, "Y"=6178439.698337167}, {"X"=4531112.978970496, "Y"=6178439.793573919}, {"X"=4531111.604831579, "Y"=6178439.764560291}, {"X"=4531110.167010706, "Y"=6178439.790818312}, {"X"=4531108.717716249, "Y"=6178439.881090899}, {"X"=4531107.251612302, "Y"=6178439.975142099}, {"X"=4531105.856218201, "Y"=6178439.899711062}, {"X"=4531104.335238762, "Y"=6178439.954901642}, {"X"=4531102.807232527, "Y"=6178440.124303117}, {"X"=4531101.328766988, "Y"=6178440.272329651}, {"X"=4531099.891838069, "Y"=6178440.308627729}, {"X"=4531098.531042268, "Y"=6178440.430204515}, {"X"=4531097.2551853685, "Y"=6178440.542927866}, {"X"=4531095.906753391, "Y"=6178440.610529815}, {"X"=4531094.453905393, "Y"=6178440.660646058}, {"X"=4531093.051487248, "Y"=6178440.699426771}, {"X"=4531091.507563893, "Y"=6178440.882646296}, {"X"=4531090.124624367, "Y"=6178440.947766378}, {"X"=4531088.636379567, "Y"=6178440.985361588}, {"X"=4531086.920802104, "Y"=6178441.166209676}, {"X"=4531085.168048208, "Y"=6178441.314457928}, {"X"=4531083.614256263, "Y"=6178441.1927222395}, {"X"=4531082.135708063, "Y"=6178441.1462256685}, {"X"=4531080.787191631, "Y"=6178441.019304884}, {"X"=4531079.550118306, "Y"=6178440.795660042}, {"X"=4531078.355558375, "Y"=6178440.664850496}, {"X"=4531077.03630355, "Y"=6178440.674700762}, {"X"=4531075.614411686, "Y"=6178440.68714403}, {"X"=4531074.112918239, "Y"=6178440.7686761385}, {"X"=4531072.594615453, "Y"=6178440.853986876}, {"X"=4531071.1807291135, "Y"=6178440.956783168}, {"X"=4531069.776626355, "Y"=6178441.170010469}, {"X"=4531068.367187707, "Y"=6178441.323002671}, {"X"=4531067.229284766, "Y"=6178441.251132974}, {"X"=4531066.229328779, "Y"=6178440.994669049}, {"X"=4531065.468266617, "Y"=6178440.725462372}, {"X"=4531065.011647067, "Y"=6178440.602842985}, {"X"=4531064.836523361, "Y"=6178440.754837769}, {"X"=4531064.734775603, "Y"=6178440.767469879}, {"X"=4531064.70204554, "Y"=6178440.7850661315}, {"X"=4531064.7259704, "Y"=6178440.861600875}, {"X"=4531064.616306829, "Y"=6178440.978403134}, {"X"=4531064.571213997, "Y"=6178441.049973729}, {"X"=4531064.4960592715, "Y"=6178441.16925804}, {"X"=4531064.430599156, "Y"=6178441.204450528}, {"X"=4531064.349218701, "Y"=6178441.253460727}, {"X"=4531064.235997578, "Y"=6178441.330106311}, {"X"=4531064.123665855, "Y"=6178441.41679105}, {"X"=4531064.026365073, "Y"=6178441.479618935}, {"X"=4531064.015781082, "Y"=6178441.553671578}, {"X"=4531064.05562626, "Y"=6178441.616388603}]
  out "Array 3":string[](array[string])=["063036.00,A,3723.59721,N,12656.92355,E,0.075,,250720,,,F,V*10", "063037.00,A,3723.59723,N,12656.92339,E,0.049,,250720,,,F,V*16", "063038.00,A,3723.59726,N,12656.92329,E,0.034,,250720,,,F,V*17", "063039.00,A,3723.59730,N,12656.92323,E,0.031,,250720,,,F,V*1E", "063040.00,A,3723.59736,N,12656.92319,E,0.013,,250720,,,F,V*1F", "063041.00,A,3723.59738,N,12656.92320,E,0.017,,250720,,,F,V*1E", "063042.00,A,3723.59738,N,12656.92319,E,0.038,,250720,,,F,V*1A", "063043.00,A,3723.59739,N,12656.92316,E,0.016,,250720,,,F,V*19", "063044.00,A,3723.59740,N,12656.92309,E,0.027,,250720,,,F,V*1C", "063045.00,A,3723.59742,N,12656.92299,E,0.034,,250720,,,F,V*15", "063046.00,A,3723.59744,N,12656.92290,E,0.024,,250720,,,F,V*18", "063047.00,A,3723.59743,N,12656.92289,E,0.027,,250720,,,F,V*15", "063048.00,A,3723.59744,N,12656.92287,E,0.037,,250720,,,F,V*12", "063049.00,A,3723.59747,N,12656.92284,E,0.045,,250720,,,F,V*16", "063112.00,A,3723.59757,N,12656.92264,E,0.063,,250720,,,A,V*15", "063113.00,A,3723.59756,N,12656.92259,E,0.036,,250720,,,A,V*1B", "063114.00,A,3723.59754,N,12656.92252,E,0.020,,250720,,,A,V*12", "063115.00,A,3723.59751,N,12656.92245,E,0.048,,250720,,,A,V*1E", "063116.00,A,3723.59748,N,12656.92239,E,0.037,,250720,,,A,V*16", "063117.00,A,3723.59745,N,12656.92231,E,0.030,,250720,,,A,V*15", "063118.00,A,3723.59738,N,12656.92228,E,0.036,,250720,,,A,V*1E", "063119.00,A,3723.59734,N,12656.92223,E,0.091,,250720,,,A,V*15", "063120.00,A,3723.59734,N,12656.92220,E,0.132,,250720,,,A,V*14", "063121.00,A,3723.59733,N,12656.92222,E,0.059,,250720,,,A,V*1C", "063122.00,A,3723.59733,N,12656.92224,E,0.013,,250720,,,A,V*17", "063123.00,A,3723.59733,N,12656.92225,E,0.115,,250720,,,A,V*10", "063124.00,A,3723.59735,N,12656.92225,E,0.025,,250720,,,A,V*13", "063125.00,A,3723.59741,N,12656.92225,E,0.065,,250720,,,A,V*15", "063126.00,A,3723.59756,N,12656.92244,E,0.046,,250720,,,A,V*16", "063127.00,A,3723.59764,N,12656.92260,E,0.050,,250720,,,A,V*17", "063128.00,A,3723.59773,N,12656.92254,E,0.079,,250720,,,A,V*12", "063129.00,A,3723.59772,N,12656.92244,E,0.012,,250720,,,A,V*1E", "063130.00,A,3723.59776,N,12656.92234,E,0.022,,250720,,,A,V*16", "063131.00,A,3723.59787,N,12656.92230,E,0.068,,250720,,,A,V*13", "063132.00,A,3723.59795,N,12656.92203,E,0.581,276.87,250720,,,A,V*03", "063133.00,A,3723.59810,N,12656.92166,E,0.706,287.68,250720,,,A,V*02", "063134.00,A,3723.59815,N,12656.92133,E,0.773,280.89,250720,,,A,V*0A", "063135.00,A,3723.59816,N,12656.92082,E,1.381,271.34,250720,,,A,V*03", "063136.00,A,3723.59815,N,12656.92024,E,1.833,271.61,250720,,,A,V*0D", "063137.00,A,3723.59812,N,12656.91931,E,2.614,271.21,250720,,,A,V*09", "063138.00,A,3723.59807,N,12656.91853,E,1.901,268.42,250720,,,A,V*02", "063139.00,A,3723.59786,N,12656.91776,E,2.418,255.02,250720,,,A,V*01", "063140.00,A,3723.59760,N,12656.91697,E,2.248,248.23,250720,,,A,V*05", "063141.00,A,3723.59727,N,12656.91638,E,2.115,244.09,250720,,,A,V*0D", "063142.00,A,3723.59695,N,12656.91567,E,2.395,244.05,250720,,,A,V*09", "063143.00,A,3723.59663,N,12656.91504,E,1.929,242.00,250720,,,A,V*09", "063144.00,A,3723.59637,N,12656.91448,E,1.677,245.59,250720,,,A,V*09", "063145.00,A,3723.59588,N,12656.91390,E,2.291,249.09,250720,,,A,V*0B", "063146.00,A,3723.59541,N,12656.91347,E,1.542,246.11,250720,,,A,V*0B", "063147.00,A,3723.59522,N,12656.91271,E,2.086,256.06,250720,,,A,V*02", "063148.00,A,3723.59509,N,12656.91213,E,1.321,255.56,250720,,,A,V*0B", "063149.00,A,3723.59498,N,12656.91145,E,1.893,261.73,250720,,,A,V*01", "063150.00,A,3723.59481,N,12656.91076,E,1.834,251.68,250720,,,A,V*04", "063151.00,A,3723.59466,N,12656.91009,E,1.823,252.04,250720,,,A,V*0B", "063152.00,A,3723.59442,N,12656.90936,E,2.413,243.69,250720,,,A,V*0D", "063153.00,A,3723.59414,N,12656.90881,E,1.687,242.24,250720,,,A,V*06", "063154.00,A,3723.59385,N,12656.90820,E,2.207,242.19,25072", "063155.00,A,3723.59354,N,12656.90741,E,2.586,244.51,250720,,,A,V*05", "063156.00,A,3723.59331,N,12656.90657,E,2.363,247.64,250720,,,A,V*0B", "063157.00,A,3723.59301,N,12656.90594,E,2.055,240.32,250720,,,A,V*07", "063158.00,A,3723.59272,N,12656.90517,E,2.516,243.46,250720,,,A,V*04", "063159.00,A,3723.59224,N,12656.90459,E,2.452,231.70,250720,,,A,V*0C", "063200.00,A,3723.59172,N,12656.90375,E,2.939,242.04,250720,,,A,V*0D", "063201.00,A,3723.59136,N,12656.90287,E,2.515,243.55,250720,,,A,V*07", "063202.00,A,3723.59100,N,12656.90217,E,2.245,246.64,250720,,,A,V*0D", "063203.00,A,3723.59066,N,12656.90141,E,2.579,245.75,250720,,,A,V*06", "063204.00,A,3723.59029,N,12656.90081,E,1.662,241.82,250720,,,A,V*01", "063205.00,A,3723.58998,N,12656.90014,E,2.136,241.99,250720,,,A,V*01", "063206.00,A,3723.58961,N,12656.89935,E,2.326,241.05,250720,,,A,V*00", "063207.00,A,3723.58933,N,12656.89844,E,2.820,250.93,250720,,,A,V*03", "063208.00,A,3723.58905,N,12656.89754,E,2.505,248.16,250720,,,A,V*09", "063209.00,A,3723.58870,N,12656.89689,E,2.550,245.90,250720,,,A,V*09", "063210.00,A,3723.58826,N,12656.89626,E,2.439,241.16,250720,,,A,V*03", "063211.00,A,3723.58792,N,12656.89554,E,2.253,244.28,250720,,,A,V*06", "063212.00,A,3723.58766,N,12656.89482,E,2.352,245.07,250720,,,A,V*08", "063213.00,A,3723.58744,N,12656.89395,E,2.491,248.96,250720,,,A,V*05", "063214.00,A,3723.58737,N,12656.89325,E,1.649,256.47,250720,,,A,V*0A", "063215.00,A,3723.58722,N,12656.89253,E,2.170,255.41,250720,,,A,V*04", "063216.00,A,3723.58705,N,12656.89185,E,1.842,256.98,250720,,,A,V*06", "063217.00,A,3723.58688,N,12656.89127,E,1.538,256.50,250720,,,A,V*0F", "063218.00,A,3723.58655,N,12656.89054,E,2.501,245.25,250720,,,A,V*0C", "063219.00,A,3723.58631,N,12656.88971,E,2.155,249.55,250720,,,A,V*0E", "063220.00,A,3723.58598,N,12656.88901,E,2.170,243.37,250720,,,A,V*0A", "063221.00,A,3723.58575,N,12656.88825,E,1.887,247.66,250720,,,A,V*0D", "063222.00,A,3723.58540,N,12656.88758,E,2.215,231.21,250720,,,A,V*0D", "063223.00,A,3723.58478,N,12656.88687,E,2.863,223.19,250720,,,A,V*06", "063224.00,A,3723.58422,N,12656.88617,E,2.497,225.12,250720,,,A,V*0D", "063225.00,A,3723.58378,N,12656.88555,E,1.879,225.45,250720,,,A,V*0C", "063226.00,A,3723.58326,N,12656.88497,E,2.303,226.01,250720,,,A,V*0D", "063227.00,A,3723.58280,N,12656.88444,E,1.970,224.59,250720,,,A,V*0D", "063228.00,A,3723.58229,N,12656.88408,E,1.830,220.56,250720,,,A,V*07", "063229.00,A,3723.58178,N,12656.88371,E,1.939,220.07,250720,,,A,V*04", "063230.00,A,3723.58137,N,12656.88339,E,1.389,222.17,250720,,,A,V*09", "063231.00,A,3723.58085,N,12656.88295,E,2.077,221.49,250720,,,A,V*0E", "063232.00,A,3723.58039,N,12656.88250,E,1.899,223.74,250720,,,A,V*04", "063233.00,A,3723.57993,N,12656.88193,E,2.317,227.60,250720,,,A,V*00", "063234.00,A,3723.57933,N,12656.88132,E,2.244,224.99,250720,,,A,V*04", "063235.00,A,3723.57879,N,12656.88082,E,2.032,222.66,250720,,,A,V*05", "063236.00,A,3723.57815,N,12656.88033,E,2.154,217.37,250720,,,A,V*05", "063237.00,A,3723.57758,N,12656.87985,E,2.286,216.12,250720,,,A,V*03", "063238.00,A,3723.57687,N,12656.87939,E,2.342,213.35,250720,,,A,V*01", "063239.00,A,3723.57633,N,12656.87904,E,1.997,209.10,250720,,,A,V*0C", "063240.00,A,3723.57564,N,12656.87873,E,2.169,207.53,250720,,,A,V*01", "063241.00,A,3723.57503,N,12656.87855,E,2.187,199.99,250720,,,A,V*07", "063242.00,A,3723.57424,N,12656.87859,E,2.435,188.33,250720,,,A,V*00", "063243.00,A,3723.57349,N,12656.87860,E,2.433,186.07,250720,,,A,V*08", "063244.00,A,3723.57270,N,12656.87856,E,2.854,182.19,250720,,,A,V*07", "063245.00,A,3723.57187,N,12656.87850,E,2.308,181.79,250720,,,A,V*0C", "063246.00,A,3723.57104,N,12656.87832,E,2.485,184.02,250720,,,A,V*0B", "063247.00,A,3723.57014,N,12656.87821,E,2.664,183.23,250720,,,A,V*01", "063248.00,A,3723.56938,N,12656.87828,E,2.535,179.88,250720,,,A,V*02", "063249.00,A,3723.56874,N,12656.87823,E,2.116,184.83,250720,,,A,V*0D", "063250.00,A,3723.56793,N,12656.87816,E,2.925,184.39,250720,,,A,V*0C", "063251.00,A,3723.56713,N,12656.87812,E,2.582,182.22,250720,,,A,V*0C", "063252.00,A,3723.56623,N,12656.87808,E,2.976,183.28,250720,,,A,V*0A", "063253.00,A,3723.56539,N,12656.87780,E,2.504,191.50,250720,,,A,V*09", "063254.00,A,3723.56458,N,12656.87773,E,2.859,189.96,250720,,,A,V*02", "063255.00,A,3723.56374,N,12656.87766,E,2.726,182.91,250720,,,A,V*05", "063256.00,A,3723.56292,N,12656.87769,E,2.473,180.38,250720,,,A,V*02", "063257.00,A,3723.56222,N,12656.87765,E,2.634,182.35,250720,,,A,V*0A", "063258.00,A,3723.56153,N,12656.87758,E,2.312,183.36,250720,,,A,V*0D", "063259.00,A,3723.56087,N,12656.87771,E,2.306,177.59,250720,,,A,V*08", "063300.00,A,3723.56019,N,12656.87810,E,2.585,165.17,250720,,,A,V*0E", "063301.00,A,3723.55957,N,12656.87829,E,2.122,169.76,250720,,,A,V*07", "063302.00,A,3723.55894,N,12656.87861,E,2.197,165.78,250720,,,A,V*0A", "063303.00,A,3723.55828,N,12656.87852,E,2.196,181.27,250720,,,A,V*0D", "063304.00,A,3723.55758,N,12656.87879,E,2.350,167.88,250720,,,A,V*0E", "063305.00,A,3723.55693,N,12656.87903,E,2.205,172.71,250720,,,A,V*06", "063306.00,A,3723.55632,N,12656.87911,E,1.877,175.99,250720,,,A,V*00", "063307.00,A,3723.55570,N,12656.87917,E,2.252,175.15,250720,,,A,V*08", "063308.00,A,3723.55524,N,12656.87947,E,1.194,169.00,250720,,,A,V*00", "063309.00,A,3723.55458,N,12656.87982,E,2.553,165.23,250720,,,A,V*03", "063310.00,A,3723.55374,N,12656.88017,E,2.314,171.10,250720,,,A,V*08", "063311.00,A,3723.55295,N,12656.88049,E,2.321,170.53,250720,,,A,V*0C", "063312.00,A,3723.55224,N,12656.88093,E,2.791,160.42,250720,,,A,V*0C", "063313.00,A,3723.55157,N,12656.88134,E,2.731,156.56,250720,,,A,V*0C", "063314.00,A,3723.55088,N,12656.88171,E,2.387,157.60,250720,,,A,V*04", "063315.00,A,3723.55037,N,12656.88217,E,2.019,152.67,250720,,,A,V*04", "063316.00,A,3723.54996,N,12656.88291,E,2.376,141.95,250720,,,A,V*0F", "063317.00,A,3723.54954,N,12656.88372,E,2.285,141.32,250720,,,A,V*0C", "063318.00,A,3723.54932,N,12656.88456,E,2.505,121.00,250720,,,A,V*0A", "063319.00,A,3723.54886,N,12656.88538,E,2.389,124.50,25072", "063320.00,A,3723.54834,N,12656.88603,E,2.440,135.96,250720,,,A,V*0E", "063321.00,A,3723.54783,N,12656.88683,E,2.732,132.03,250720,,,A,V*09", "063322.00,A,3723.54735,N,12656.88769,E,2.827,129.18,250720,,,A,V*09", "063323.00,A,3723.54684,N,12656.88847,E,2.455,134.48,250720,,,A,V*00", "063324.00,A,3723.54636,N,12656.88906,E,2.333,135.24,250720,,,A,V*06", "063325.00,A,3723.54576,N,12656.88963,E,2.269,131.77,250720,,,A,V*0F", "063326.00,A,3723.54521,N,12656.89029,E,2.243,131.25,250720,,,A,V*07", "063327.00,A,3723.54462,N,12656.89091,E,2.448,131.91,250720,,,A,V*01", "063328.00,A,3723.54406,N,12656.89149,E,2.374,133.71,250720,,,A,V*0C", "063329.00,A,3723.54358,N,12656.89203,E,2.258,133.54,250720,,,A,V*04", "063330.00,A,3723.54309,N,12656.89278,E,2.571,125.19,250720,,,A,V*06", "063331.00,A,3723.54247,N,12656.89342,E,2.522,131.21,25072", "063332.00,A,3723.54183,N,12656.89398,E,2.531,136.97,250720,,,A,V*0B", "063333.00,A,3723.54121,N,12656.89454,E,2.481,135.92,250720,,,A,V*09", "063334.00,A,3723.54077,N,12656.89504,E,2.149,138.68,250720,,,A,V*01", "063335.00,A,3723.54025,N,12656.89560,E,2.568,137.87,250720,,,A,V*0C", "063336.00,A,3723.53973,N,12656.89622,E,2.521,141.20,250720,,,A,V*06", "063337.00,A,3723.53911,N,12656.89657,E,2.149,148.95,250720,,,A,V*0C", "063338.00,A,3723.53849,N,12656.89702,E,2.327,142.00,250720,,,A,V*02", "063339.00,A,3723.53801,N,12656.89766,E,2.418,137.85,250720,,,A,V*09", "063340.00,A,3723.53740,N,12656.89821,E,2.583,140.58,250720,,,A,V*02", "063341.00,A,3723.53673,N,12656.89858,E,2.511,155.60,250720,,,A,V*08", "063342.00,A,3723.53624,N,12656.89906,E,2.072,146.01,250720,,,A,V*06", "063343.00,A,3723.53575,N,12656.89962,E,2.428,139.12,250720,,,A,V*03", "063344.00,A,3723.53511,N,12656.90024,E,2.736,139.55,250720,,,A,V*0A", "063345.00,A,3723.53453,N,12656.90083,E,2.353,141.28,250720,,,A,V*03", "063346.00,A,3723.53407,N,12656.90136,E,1.928,136.50,250720,,,A,V*04", "063347.00,A,3723.53356,N,12656.90170,E,1.863,143.41,250720,,,A,V*08", "063348.00,A,3723.53299,N,12656.90210,E,2.178,142.93,250720,,,A,V*0E", "063349.00,A,3723.53259,N,12656.90253,E,1.685,140.86,250720,,,A,V*04", "063350.00,A,3723.53204,N,12656.90303,E,2.318,141.72,250720,,,A,V*08", "063351.00,A,3723.53133,N,12656.90334,E,2.085,146.06,250720,,,A,V*09", "063352.00,A,3723.53070,N,12656.90384,E,2.386,144.20,250720,,,A,V*01", "063353.00,A,3723.53011,N,12656.90440,E,2.479,142.48,250720,,,A,V*07", "063354.00,A,3723.52964,N,12656.90504,E,2.172,138.50,250720,,,A,V*01", "063355.00,A,3723.52908,N,12656.90537,E,2.173,148.73,250720,,,A,V*0D", "063356.00,A,3723.52851,N,12656.90592,E,2.546,143.70,250720,,,A,V*06", "063357.00,A,3723.52791,N,12656.90655,E,2.423,141.33,250720,,,A,V*0B", "063358.00,A,3723.52738,N,12656.90726,E,2.492,134.18,250720,,,A,V*03", "063359.00,A,3723.52682,N,12656.90785,E,2.526,136.35,250720,,,A,V*08", "063400.00,A,3723.52626,N,12656.90848,E,2.283,137.30,250720,,,A,V*0F", "063401.00,A,3723.52582,N,12656.90897,E,1.920,138.51,250720,,,A,V*08", "063402.00,A,3723.52530,N,12656.90960,E,2.276,140.56,250720,,,A,V*08", "063403.00,A,3723.52476,N,12656.91012,E,2.235,140.88,250720,,,A,V*03", "063404.00,A,3723.52444,N,12656.91092,E,2.406,118.96,250720,,,A,V*09", "063405.00,A,3723.52421,N,12656.91187,E,2.549,108.18,250720,,,A,V*03", "063406.00,A,3723.52402,N,12656.91285,E,2.881,105.10,250720,,,A,V*0C", "063407.00,A,3723.52395,N,12656.91374,E,2.249,97.97,250720,,,A,V*30", "063408.00,A,3723.52388,N,12656.91461,E,2.047,100.55,250720,,,A,V*0D", "063409.00,A,3723.52390,N,12656.91536,E,2.344,89.27,250720,,,A,V*33", "063410.00,A,3723.52394,N,12656.91630,E,2.260,82.97,250720,,,A,V*3D", "063411.00,A,3723.52410,N,12656.91707,E,1.940,77.66,250720,,,A,V*3C", "063412.00,A,3723.52439,N,12656.91797,E,2.482,61.01,250720,,,A,V*3B", "063413.00,A,3723.52465,N,12656.91881,E,2.199,65.08,250720,,,A,V*39", "063414.00,A,3723.52486,N,12656.91960,E,2.297,66.68,250720,,,A,V*35", "063415.00,A,3723.52522,N,12656.92028,E,2.433,56.07,250720,,,A,V*3F", "063416.00,A,3723.52561,N,12656.92100,E,2.472,56.88,250720,,,A,V*32", "063417.00,A,3723.52608,N,12656.92170,E,2.644,49.87,250720,,,A,V*3E", "063418.00,A,3723.52646,N,12656.92232,E,1.859,50.75,250720,,,A,V*3A", "063419.00,A,3723.52687,N,12656.92293,E,2.273,47.62,250720,,,A,V*3C", "063420.00,A,3723.52728,N,12656.92367,E,2.440,56.03,250720,,,A,V*39", "063421.00,A,3723.52776,N,12656.92447,E,2.736,54.22,250720,,,A,V*35", "063422.00,A,3723.52821,N,12656.92517,E,2.555,50.98,250720,,,A,V*3D", "063423.00,A,3723.52868,N,12656.92593,E,2.834,52.22,250720,,,A,V*34", "063424.00,A,3723.52907,N,12656.92659,E,2.354,51.87,250720,,,A,V*3F", "063425.00,A,3723.52955,N,12656.92725,E,2.592,48.70,250720,,,A,V*3F", "063426.00,A,3723.53011,N,12656.92797,E,2.831,46.52,250720,,,A,V*37", "063427.00,A,3723.53052,N,12656.92867,E,2.361,51.02,250720,,,A,V*3C", "063428.00,A,3723.53092,N,12656.92937,E,2.429,52.54,250720,,,A,V*30", "063429.00,A,3723.53137,N,12656.93005,E,2.307,54.54,250720,,,A,V*3B", "063430.00,A,3723.53180,N,12656.93075,E,2.429,57.64,250720,,,A,V*33", "063431.00,A,3723.53237,N,12656.93141,E,2.695,48.29,250720,,,A,V*39", "063432.00,A,3723.53295,N,12656.93208,E,2.638,47.91,250720,,,A,V*37", "063433.00,A,3723.53353,N,12656.93272,E,2.618,46.97,250720,,,A,V*35", "063434.00,A,3723.53397,N,12656.93344,E,2.426,52.57,250720,,,A,V*38", "063435.00,A,3723.53446,N,12656.93412,E,2.575,51.06,250720,,,A,V*36", "063436.00,A,3723.53494,N,12656.93480,E,2.439,51.72,250720,,,A,V*3B", "063437.00,A,3723.53524,N,12656.93553,E,2.179,63.28,250720,,,A,V*30", "063438.00,A,3723.53570,N,12656.93630,E,2.500,60.43,250720,,,A,V*3C", "063439.00,A,3723.53624,N,12656.93705,E,2.710,54.59,250720,,,A,V*37", "063440.00,A,3723.53672,N,12656.93780,E,2.553,54.72,250720,,,A,V*3B", "063441.00,A,3723.53718,N,12656.93863,E,2.778,58.01,250720,,,A,V*36", "063442.00,A,3723.53770,N,12656.93935,E,2.697,52.97,250720,,,A,V*3C", "063443.00,A,3723.53832,N,12656.94006,E,2.708,50.79,250720,,,A,V*3F", "063444.00,A,3723.53886,N,12656.94071,E,2.269,50.47,250720,,,A,V*38", "063445.00,A,3723.53934,N,12656.94136,E,2.268,53.19,250720,,,A,V*3A", "063446.00,A,3723.53988,N,12656.94182,E,1.674,54.41,250720,,,A,V*31", "063447.00,A,3723.54055,N,12656.94207,E,1.731,41.35,250720,,,A,V*37", "063448.00,A,3723.54099,N,12656.94261,E,2.225,42.65,250720,,,A,V*3D", "063449.00,A,3723.54141,N,12656.94344,E,2.524,53.32,250720,,,A,V*3A", "063450.00,A,3723.54195,N,12656.94427,E,2.759,55.61,250720,,,A,V*31", "063451.00,A,3723.54255,N,12656.94501,E,2.525,47.16,250720,,,A,V*30", "063452.00,A,3723.54299,N,12656.94574,E,2.338,56.82,250720,,,A,V*36", "063453.00,A,3723.54334,N,12656.94644,E,2.204,59.86,250720,,,A,V*34", "063454.00,A,3723.54389,N,12656.94694,E,1.972,53.62,250720,,,A,V*31", "063455.00,A,3723.54442,N,12656.94750,E,2.268,53.02,250720,,,A,V*3C", "063456.00,A,3723.54500,N,12656.94833,E,2.872,52.96,250720,,,A,V*3F", "063457.00,A,3723.54542,N,12656.94904,E,2.119,54.16,250720,,,A,V*37", "063458.00,A,3723.54582,N,12656.94975,E,2.384,56.21,250720,,,A,V*32", "063459.00,A,3723.54624,N,12656.95049,E,2.345,53.94,250720,,,A,V*3D", "063500.00,A,3723.54667,N,12656.95131,E,2.514,56.26,250720,,,A,V*37", "063501.00,A,3723.54714,N,12656.95198,E,2.027,49.26,250720,,,A,V*3B", "063502.00,A,3723.54749,N,12656.95254,E,1.694,58.38,250720,,,A,V*31", "063503.00,A,3723.54794,N,12656.95320,E,2.212,46.60,250720,,,A,V*39", "063504.00,A,3723.54846,N,12656.95421,E,3.284,48.96,250720,,,A,V*31", "063505.00,A,3723.54869,N,12656.95532,E,2.338,55.45,250720,,,A,V*3B", "063506.00,A,3723.54895,N,12656.95641,E,2.921,64.28,250720,,,A,V*37", "063507.00,A,3723.54917,N,12656.95759,E,2.755,67.25,250720,,,A,V*36", "063508.00,A,3723.54940,N,12656.95869,E,2.892,69.17,250720,,,A,V*3C", "063509.00,A,3723.54963,N,12656.95971,E,2.819,71.56,250720,,,A,V*3B", "063510.00,A,3723.54988,N,12656.96063,E,2.355,69.45,250720,,,A,V*37", "063511.00,A,3723.55015,N,12656.96165,E,2.879,69.97,250720,,,A,V*37", "063512.00,A,3723.55032,N,12656.96280,E,3.055,75.42,250720,,,A,V*3B", "063513.00,A,3723.55054,N,12656.96368,E,2.156,74.18,250720,,,A,V*30", "063514.00,A,3723.55085,N,12656.96451,E,2.470,69.95,250720,,,A,V*3E", "063515.00,A,3723.55109,N,12656.96527,E,2.136,70.77,250720,,,A,V*39", "063516.00,A,3723.55125,N,12656.96584,E,1.313,71.51,250720,,,A,V*3E", "063517.00,A,3723.55152,N,12656.96674,E,2.773,69.66,250720,,,A,V*3F", "063518.00,A,3723.55174,N,12656.96744,E,1.803,70.50,250720,,,A,V*30", "063519.00,A,3723.55220,N,12656.96800,E,2.159,56.53,250720,,,A,V*3E", "063520.00,A,3723.55250,N,12656.96883,E,2.553,64.84,250720,,,A,V*3D", "063521.00,A,3723.55291,N,12656.96958,E,2.115,54.32,250720,,,A,V*3E", "063522.00,A,3723.55337,N,12656.97015,E,2.210,53.41,250720,,,A,V*34", "063523.00,A,3723.55374,N,12656.97090,E,2.221,60.05,250720,,,A,V*3D", "063524.00,A,3723.55410,N,12656.97164,E,2.179,58.98,250720,,,A,V*34", "063525.00,A,3723.55453,N,12656.97234,E,2.134,60.62,250720,,,A,V*33", "063526.00,A,3723.55483,N,12656.97299,E,1.995,66.69,250720,,,A,V*37", "063527.00,A,3723.55512,N,12656.97373,E,1.980,64.93,250720,,,A,V*39", "063528.00,A,3723.55551,N,12656.97460,E,2.763,62.19,250720,,,A,V*30", "063529.00,A,3723.55588,N,12656.97552,E,2.784,64.78,250720,,,A,V*3D", "063530.00,A,3723.55617,N,12656.97636,E,1.905,68.30,250720,,,A,V*35", "063531.00,A,3723.55660,N,12656.97735,E,2.764,65.93,250720,,,A,V*38", "063532.00,A,3723.55693,N,12656.97827,E,2.289,69.66,250720,,,A,V*3B", "063533.00,A,3723.55720,N,12656.97898,E,1.729,69.61,250720,,,A,V*3C", "063534.00,A,3723.55755,N,12656.97987,E,2.604,63.43,250720,,,A,V*31", "063535.00,A,3723.55770,N,12656.98083,E,2.147,69.59,250720,,,A,V*34", "063536.00,A,3723.55811,N,12656.98179,E,2.761,70.26,250720,,,A,V*39", "063537.00,A,3723.55851,N,12656.98309,E,2.670,70.44,250720,,,A,V*3C", "063538.00,A,3723.55886,N,12656.98396,E,2.133,63.17,250720,,,A,V*3B", "063539.00,A,3723.55943,N,12656.98469,E,2.401,57.28,250720,,,A,V*3A", "063540.00,A,3723.55992,N,12656.98548,E,2.112,55.85,250720,,,A,V*38", "063541.00,A,3723.56042,N,12656.98646,E,2.664,46.56,250720,,,A,V*39", "063542.00,A,3723.56105,N,12656.98731,E,3.030,45.73,250720,,,A,V*3B", "063543.00,A,3723.56157,N,12656.98811,E,2.443,48.56,250720,,,A,V*3B", "063544.00,A,3723.56191,N,12656.98917,E,2.911,55.26,250720,,,A,V*30", "063545.00,A,3723.56241,N,12656.98992,E,2.057,48.45,250720,,,A,V*30", "063546.00,A,3723.56277,N,12656.99019,E,0.878,39.57,250720,,,A,V*3F", "063547.00,A,3723.56318,N,12656.99062,E,1.907,31.26,250720,,,A,V*3C", "063548.00,A,3723.56384,N,12656.99088,E,2.327,18.77,250720,,,A,V*36", "063549.00,A,3723.56461,N,12656.99152,E,3.081,20.58,250720,,,A,V*35", "063550.00,A,3723.56521,N,12656.99230,E,2.609,28.20,250720,,,A,V*3F", "063551.00,A,3723.56566,N,12656.99291,E,1.383,29.83,250720,,,A,V*3A", "063552.00,A,3723.56605,N,12656.99302,E,1.745,13.10,250720,,,A,V*39", "063553.00,A,3723.56657,N,12656.99294,E,2.490,354.25,250720,,,A,V*0F", "063554.00,A,3723.56712,N,12656.99262,E,2.641,335.19,250720,,,A,V*07", "063555.00,A,3723.56782,N,12656.99245,E,2.908,342.11,250720,,,A,V*00", "063556.00,A,3723.56845,N,12656.99182,E,3.527,325.19,250720,,,A,V*06", "063557.00,A,3723.56894,N,12656.99146,E,1.999,330.89,250720,,,A,V*05", "063558.00,A,3723.56961,N,12656.99123,E,2.435,339.49,250720,,,A,V*0F", "063559.00,A,3723.57022,N,12656.99091,E,2.270,338.80,250720,,,A,V*0A", "063600.00,A,3723.57083,N,12656.99059,E,2.289,340.76,250720,,,A,V*0A", "063601.00,A,3723.57137,N,12656.99058,E,1.528,345.50,250720,,,A,V*0A", "063602.00,A,3723.57192,N,12656.99065,E,2.154,345.92,250720,,,A,V*0A", "063603.00,A,3723.57249,N,12656.99042,E,2.037,341.93,250720,,,A,V*0A", "063604.00,A,3723.57304,N,12656.99015,E,1.963,339.85,250720,,,A,V*04", "063605.00,A,3723.57369,N,12656.99011,E,2.188,352.14,250720,,,A,V*01", "063606.00,A,3723.57431,N,12656.98981,E,2.427,334.30,250720,,,A,V*0F", "063607.00,A,3723.57495,N,12656.98923,E,2.620,328.22,250720,,,A,V*03", "063608.00,A,3723.57562,N,12656.98893,E,2.510,337.50,250720,,,A,V*04", "063609.00,A,3723.57619,N,12656.98861,E,1.881,334.15,250720,,,A,V*03", "063610.00,A,3723.57673,N,12656.98841,E,1.868,341.20,250720,,,A,V*06", "063611.00,A,3723.57739,N,12656.98808,E,2.222,333.07,250720,,,A,V*02", "063612.00,A,3723.57803,N,12656.98783,E,2.300,339.52,250720,,,A,V*00", "063613.00,A,3723.57848,N,12656.98770,E,1.114,340.38,250720,,,A,V*04", "063614.00,A,3723.57902,N,12656.98740,E,1.999,337.63,250720,,,A,V*0C", "063615.00,A,3723.57965,N,12656.98709,E,2.058,337.44,250720,,,A,V*03", "063616.00,A,3723.58027,N,12656.98687,E,1.932,339.09,250720,,,A,V*06", "063617.00,A,3723.58085,N,12656.98663,E,1.703,336.46,250720,,,A,V*0D", "063618.00,A,3723.58130,N,12656.98626,E,1.720,328.09,250720,,,A,V*09", "063619.00,A,3723.58168,N,12656.98575,E,2.058,312.19,250720,,,A,V*03", "063620.00,A,3723.58226,N,12656.98534,E,2.217,323.88,250720,,,A,V*06", "063621.00,A,3723.58269,N,12656.98502,E,0.832,321.19,250720,,,A,V*0C", "063622.00,A,3723.58328,N,12656.98482,E,2.184,332.29,250720,,,A,V*05", "063623.00,A,3723.58386,N,12656.98459,E,1.578,338.85,250720,,,A,V*0E", "063624.00,A,3723.58446,N,12656.98450,E,1.768,344.33,250720,,,A,V*0E", "063625.00,A,3723.58504,N,12656.98434,E,1.626,343.02,250720,,,A,V*04", "063626.00,A,3723.58545,N,12656.98397,E,1.598,332.49,250720,,,A,V*03", "063627.00,A,3723.58609,N,12656.98366,E,2.062,341.26,250720,,,A,V*09", "063628.00,A,3723.58680,N,12656.98346,E,2.208,349.66,250720,,,A,V*07", "063629.00,A,3723.58752,N,12656.98312,E,2.122,345.50,250720,,,A,V*0B", "063630.00,A,3723.58818,N,12656.98270,E,2.191,339.03,250720,,,A,V*02", "063631.00,A,3723.58877,N,12656.98228,E,1.952,334.60,250720,,,A,V*0B", "063632.00,A,3723.58939,N,12656.98185,E,1.933,333.80,250720,,,A,V*09", "063633.00,A,3723.59017,N,12656.98170,E,2.281,345.20,250720,,,A,V*0C", "063634.00,A,3723.59083,N,12656.98137,E,2.261,343.71,250720,,,A,V*09", "063635.00,A,3723.59160,N,12656.98099,E,1.772,345.73,250720,,,A,V*01", "063636.00,A,3723.59229,N,12656.98073,E,2.332,343.82,250720,,,A,V*03", "063637.00,A,3723.59314,N,12656.98034,E,2.701,337.92,250720,,,A,V*08", "063638.00,A,3723.59395,N,12656.97979,E,2.796,334.42,250720,,,A,V*01", "063639.00,A,3723.59481,N,12656.97950,E,2.529,342.27,250720,,,A,V*0D", "063640.00,A,3723.59557,N,12656.97924,E,2.272,340.66,250720,,,A,V*04", "063641.00,A,3723.59624,N,12656.97889,E,2.446,340.31,250720,,,A,V*07", "063642.00,A,3723.59694,N,12656.97836,E,2.540,329.01,250720,,,A,V*00", "063643.00,A,3723.59757,N,12656.97803,E,2.272,335.65,250720,,,A,V*00", "063644.00,A,3723.59833,N,12656.97773,E,2.390,338.75,250720,,,A,V*03", "063645.00,A,3723.59911,N,12656.97748,E,2.191,340.66,250720,,,A,V*05", "063646.00,A,3723.59979,N,12656.97713,E,2.413,337.23,250720,,,A,V*08", "063647.00,A,3723.60050,N,12656.97668,E,2.659,332.32,250720,,,A,V*05", "063648.00,A,3723.60125,N,12656.97620,E,2.611,334.10,250720,,,A,V*0F", "063649.00,A,3723.60191,N,12656.97552,E,2.696,324.78,250720,,,A,V*07", "063650.00,A,3723.60265,N,12656.97511,E,2.534,336.90,250720,,,A,V*0E", "063651.00,A,3723.60331,N,12656.97466,E,2.322,329.15,250720,,,A,V*0C", "063652.00,A,3723.60405,N,12656.97426,E,2.517,331.54,250720,,,A,V*07", "063653.00,A,3723.60478,N,12656.97398,E,2.397,338.03,250720,,,A,V*0B", "063654.00,A,3723.60565,N,12656.97378,E,2.839,344.20,250720,,,A,V*0A", "063655.00,A,3723.60635,N,12656.97354,E,1.810,343.05,250720,,,A,V*0B", "063656.00,A,3723.60692,N,12656.97328,E,2.057,341.59,250720,,,A,V*0D", "063657.00,A,3723.60743,N,12656.97278,E,1.885,325.59,250720,,,A,V*03", "063658.00,A,3723.60815,N,12656.97237,E,2.612,332.30,250720,,,A,V*01", "063659.00,A,3723.60894,N,12656.97198,E,2.310,334.54,250720,,,A,V*0C", "063700.00,A,3723.60949,N,12656.97138,E,2.282,321.60,250720,,,A,V*03", "063701.00,A,3723.60967,N,12656.97069,E,1.855,301.24,250720,,,A,V*0A", "063702.00,A,3723.60977,N,12656.96994,E,2.123,279.02,250720,,,A,V*03", "063703.00,A,3723.60984,N,12656.96894,E,3.098,267.29,250720,,,A,V*09", "063704.00,A,3723.60982,N,12656.96803,E,2.391,266.63,250720,,,A,V*02", "063705.00,A,3723.60973,N,12656.96723,E,2.386,259.76,250720,,,A,V*0E", "063706.00,A,3723.60962,N,12656.96641,E,2.473,254.26,250720,,,A,V*0D", "063707.00,A,3723.60943,N,12656.96570,E,2.130,249.62,250720,,,A,V*00", "063708.00,A,3723.60927,N,12656.96492,E,2.516,249.89,250720,,,A,V*05", "063709.00,A,3723.60912,N,12656.96401,E,2.684,253.89,250720,,,A,V*0B", "063710.00,A,3723.60889,N,12656.96307,E,2.763,247.30,250720,,,A,V*0E", "063711.00,A,3723.60873,N,12656.96210,E,3.026,256.90,250720,,,A,V*00", "063712.00,A,3723.60841,N,12656.96127,E,2.845,244.86,250720,,,A,V*0D", "063713.00,A,3723.60819,N,12656.96043,E,2.543,246.92,250720,,,A,V*0E", "063714.00,A,3723.60805,N,12656.95975,E,1.913,249.33,250720,,,A,V*05", "063715.00,A,3723.60775,N,12656.95888,E,2.991,244.44,250720,,,A,V*0B", "063716.00,A,3723.60739,N,12656.95798,E,2.717,241.82,250720,,,A,V*01", "063717.00,A,3723.60715,N,12656.95718,E,2.312,244.70,250720,,,A,V*0F", "063718.00,A,3723.60706,N,12656.95629,E,2.650,255.60,250720,,,A,V*03", "063719.00,A,3723.60678,N,12656.95538,E,2.809,246.20,250720,,,A,V*0D", "063720.00,A,3723.60661,N,12656.95458,E,2.327,249.45,250720,,,A,V*03", "063721.00,A,3723.60640,N,12656.95377,E,2.522,247.51,250720,,,A,V*03", "063722.00,A,3723.60607,N,12656.95297,E,2.729,241.42,250720,,,A,V*01", "063723.00,A,3723.60578,N,12656.95213,E,2.660,245.29,250720,,,A,V*02", "063724.00,A,3723.60555,N,12656.95128,E,2.598,246.23,250720,,,A,V*0C", "063725.00,A,3723.60532,N,12656.95042,E,2.594,244.26,250720,,,A,V*0A", "063726.00,A,3723.60494,N,12656.94961,E,2.633,244.78,250720,,,A,V*08", "063727.00,A,3723.60466,N,12656.94872,E,2.739,246.24,250720,,,A,V*07", "063728.00,A,3723.60449,N,12656.94782,E,2.552,249.49,250720,,,A,V*0E", "063729.00,A,3723.60431,N,12656.94695,E,2.558,251.67,250720,,,A,V*08", "063730.00,A,3723.60403,N,12656.94611,E,2.628,250.66,250720,,,A,V*09", "063731.00,A,3723.60385,N,12656.94531,E,2.306,251.29,250720,,,A,V*03", "063732.00,A,3723.60368,N,12656.94456,E,2.059,248.08,250720,,,A,V*01", "063733.00,A,3723.60345,N,12656.94377,E,2.403,249.45,250720,,,A,V*08", "063734.00,A,3723.60318,N,12656.94292,E,2.503,246.59,250720,,,A,V*0E", "063735.00,A,3723.60291,N,12656.94210,E,2.363,244.85,250720,,,A,V*06", "063736.00,A,3723.60275,N,12656.94119,E,2.545,248.38,250720,,,A,V*0D", "063737.00,A,3723.60251,N,12656.94038,E,2.320,244.70,250720,,,A,V*0D", "063738.00,A,3723.60222,N,12656.93951,E,2.747,247.24,250720,,,A,V*00", "063739.00,A,3723.60202,N,12656.93850,E,2.799,248.44,250720,,,A,V*09", "063740.00,A,3723.60178,N,12656.93747,E,2.843,247.24,250720,,,A,V*01", "063741.00,A,3723.60132,N,12656.93657,E,2.968,243.53,250720,,,A,V*02", "063742.00,A,3723.60095,N,12656.93571,E,2.671,240.93,250720,,,A,V*02", "063743.00,A,3723.60053,N,12656.93493,E,2.590,240.72,250720,,,A,V*07", "063744.00,A,3723.60004,N,12656.93422,E,2.602,242.74,250720,,,A,V*04", "063745.00,A,3723.59965,N,12656.93353,E,2.361,241.88,250720,,,A,V*00", "063746.00,A,3723.59937,N,12656.93276,E,2.344,242.73,250720,,,A,V*02", "063747.00,A,3723.59907,N,12656.93193,E,2.536,243.40,250720,,,A,V*0A", "063748.00,A,3723.59882,N,12656.93105,E,2.616,244.84,250720,,,A,V*08", "063749.00,A,3723.59857,N,12656.93016,E,2.674,246.89,250720,,,A,V*09", "063750.00,A,3723.59836,N,12656.92933,E,2.365,249.77,250720,,,A,V*02", "063751.00,A,3723.59826,N,12656.92850,E,2.346,255.11,250720,,,A,V*0A", "063752.00,A,3723.59810,N,12656.92767,E,2.348,253.51,250720,,,A,V*0B", "063753.00,A,3723.59778,N,12656.92701,E,2.065,246.47,250720,,,A,V*04", "063754.00,A,3723.59731,N,12656.92644,E,2.385,229.80,250720,,,A,V*01", "063755.00,A,3723.59688,N,12656.92601,E,1.672,225.75,250720,,,A,V*0A", "063756.00,A,3723.59666,N,12656.92575,E,0.811,229.39,250720,,,A,V*07", "063757.00,A,3723.59677,N,12656.92564,E,0.185,,250720,,,A,V*1F", "063758.00,A,3723.59676,N,12656.92558,E,0.054,,250720,,,A,V*13", "063759.00,A,3723.59677,N,12656.92556,E,0.061,,250720,,,A,V*1B", "063800.00,A,3723.59685,N,12656.92557,E,0.038,,250720,,,A,V*18", "063801.00,A,3723.59694,N,12656.92550,E,0.023,,250720,,,A,V*14", "063802.00,A,3723.59700,N,12656.92547,E,0.021,,250720,,,A,V*1F", "063803.00,A,3723.59710,N,12656.92542,E,0.005,,250720,,,A,V*1C", "063804.00,A,3723.59712,N,12656.92538,E,0.026,,250720,,,A,V*15", "063805.00,A,3723.59715,N,12656.92533,E,0.020,,250720,,,A,V*1E", "063806.00,A,3723.59720,N,12656.92526,E,0.001,,250720,,,A,V*1C", "063807.00,A,3723.59726,N,12656.92519,E,0.043,,250720,,,A,V*11", "063808.00,A,3723.59730,N,12656.92513,E,0.012,,250720,,,A,V*17", "063809.00,A,3723.59737,N,12656.92512,E,0.021,,250720,,,A,V*10", "063810.00,A,3723.59744,N,12656.92514,E,0.024,,250720,,,A,V*1F"]
  in  "match str":string="GNRMC,"
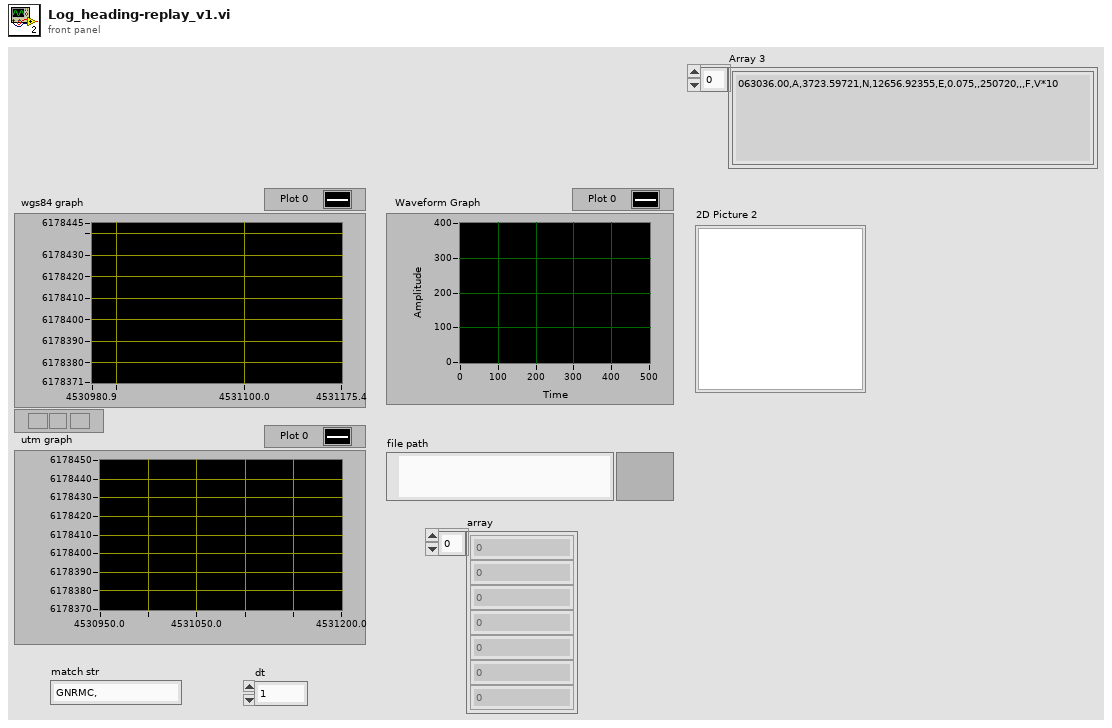
[diagram p1: front panel]
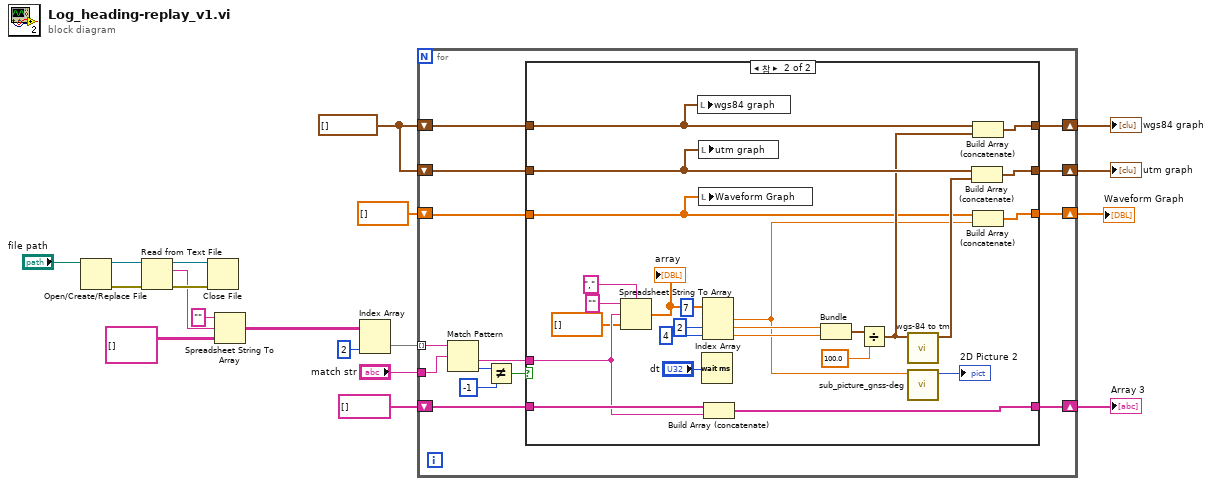
[diagram p0: block diagram]
diagram:
  w5 = cluster{dbl, dbl}[] []
  n1 = Open/Create/Replace File(file path (use dialog)="file path") -> (refnum out=w16:refnum<file>, error out=w19:errorcluster)  [unwired: 5 in, 1 out]
  n2 = Read from Text File(file (use dialog)=w16, error in=w19) -> (refnum out=w17:refnum<file>, text=w6:string, error out=w18:errorcluster)  [unwired: 2 in, 1 out]
  n3 = Close File(refnum=w17, error in=w18) -> ()  [unwired: 2 out]
  n4 = Spreadsheet String To Array(format string="", spreadsheet string=w6, array type (2D Dbl)=string[][] []) -> (array=w13:string[][])  [unwired: 1 in]
  n5 = Index Array(array=w13, index (col)=2 ("disabled index (col)")) -> (element=w11:string[])  [unwired: 1 in]
  n6 = for {
    tunnel: w11 -> [w33] mode=indexing
    tunnel: "match str" -> [w32]
    shift-right: [w27] -> w8
    shift-left: string[] [] -> [w28]
    shift-right: [w26] -> w7
    shift-left: w5 -> [w25]
    shift-right: [w22] -> w4
    shift-left: w5 -> [w23]
    shift-right: [w21] -> w2
    shift-left: dbl[] [] -> [w20]
    n7 = Match Pattern(string=w33, regular expression=w32) -> (after substring=w24:string, offset past match=w31:i32)  [unwired: 1 in, 2 out]
    n8 = Not Equal?(x=w31, y=-1) -> (x != y?=w29:bool)
    n9 = case shown="참" w29 {
      tunnel: w28 -> [w37 w62]
      tunnel: [w37 w61] -> w27
      tunnel: w24 -> [_ w55]
      tunnel: [w36 w47] -> w26
      tunnel: w25 -> [w36 w46]
      tunnel: w23 -> [w35 w43]
      tunnel: [w35 w44] -> w22
      tunnel: [w34 w41] -> w21
      tunnel: w20 -> [w34 w40]
      frame False {
      }
      frame True {
        n10 = Spreadsheet String To Array(delimiter (Tab)=",", format string="", spreadsheet string=w55, array type (2D Dbl)=dbl[] []) -> (array=w52:dbl[])
        "array" <- w52
        n11 = local write "wgs84 graph"(w43) -> ()
        n12 = local write "utm graph"(w46) -> ()
        n13 = local write "Waveform Graph"(w40) -> ()
        n14 = Wait (ms)(milliseconds to wait="dt") -> ()  [unwired: 1 out]
        n15 = Index Array(array=w52, index #1=7 ("index"), index #2=2 ("index"), index #3=4 ("index")) -> (element #1=w38:dbl, element #2=w51:dbl, element #3=w50:dbl)
        n16 = Build Array (concatenate)(w62, w55) -> (w61:string[])
        n17 = Bundle(w51, w50) -> (w59:cluster{dbl, dbl})  [unwired: 1 in]
        n18 = Divide(x=w59, y=100.0) -> (x/y=w45:cluster{dbl, dbl})
        n19 = call "wgs-84 to tm.vi"("in_lon-lat"=w45) -> ("TM"=w49:cluster{"Y(E)":dbl, "X(N)":dbl})  [unwired: 10 in]
        n20 = call "sub_picture_gnss-deg.vi"("deg_gps"=w38) -> ("new picture"=→"2D Picture 2":picture)  [unwired: 10 in]
        n21 = Build Array (concatenate)(w46, w49) -> (w47:cluster{"Y(E)":dbl, "X(N)":dbl}[])
        n22 = Build Array (concatenate)(w43, w45) -> (w44:cluster{dbl, dbl}[])
        n23 = Build Array (concatenate)(w40, w38) -> (w41:dbl[])
      }
    }
  }
  "Array 3" <- w8
  "utm graph" <- w7
  "wgs84 graph" <- w4
  "Waveform Graph" <- w2
